vi "UI Interface.vi"(8 "error in (no error)":errorcluster, 10 "GRR Results":T1[](array[typedef]), 11 "Test Data":T2[](array[typedef])) -> (0 "error out":errorcluster)   [LabVIEW 2018, in "Result Display.lvclass"]
uses:
  Result Display.lvclass
  TestDataMgr/Typedefs/Test Data All.ctl
  TestDataMgr/Typedefs/Test Limits.ctl
  TestDataMgr/Typedefs/Test Raw Data.ctl
  Result Data Mgr/Typedefs/GRR Result.ctl
  <vilib>/Utility/error.llb/Error Cluster From Error Code.vi
  <vilib>/ErrorRing/Error Ring.xnode
  TestDataMgr/TestDataMgr.lvclass
  Result Data Mgr/Result Data Mgr.lvclass
panel:
  in  "DUT Plot Visible?  DUT# 0-N":bool[](array[boolean])
  in  "stop":bool
  out "GRR Result":T1
  out "Tester#2":dbl[][](graph)
  out "Tester#1":dbl[][](graph)
  in  "Test Items":u16(ring) items=["TXV_PS_Gmax_24p25G_V4_PhaseRange", "OS_VDD_SPI_CS", "TXV_PS_Gmax_27p5G_V0_GainDelta", "TXV_PS_Gmax_29p5G_V1_PhaseRange", "TXV_GS_Phase_Dynamic_FE_24p25G_V4", "RXV_PS_Gmax_26p5G_V1_PhaseRange", "TXV_PAE_12dBm_Pout_24p25G_V3", "TXV_PD_10dBm_Vout_24p25_V1", "TXV_PS_Gmax_24p25G_V5_GainDelta", "OS_VDD_SPI_CLK_IN", "TXV_PS_Gmax_27p5G_V0_GainRMS", "TXV_PS_Gmax_29p5G_V2_GainDelta", "TXV_GS_Gain_Gmax_COM127_FE127_24p25G_V5", "RXV_PS_Gmax_26p5G_V2_GainDelta", "TXV_PAE_12dBm_PAE_24p25G_V3", "TXV_PD_15dBm_Pout_24p25_V1", "TXV_PS_Gmax_24p25G_V5_GainRMS", "OS_VDD_SPI_DATA_IN", "TXV_PS_Gmax_27p5G_V0_PhaseRange", "TXV_PS_Gmax_29p5G_V2_GainRMS", "TXV_GS_Gain_Dynamic_COM_24p25G_V5", "RXV_PS_Gmax_26p5G_V2_GainRMS", "TXV_PAE_12dBm_Pout_24p25G_V4", "TXV_PD_15dBm_Vout_24p25_V1", "TXV_PS_Gmax_24p25G_V5_PhaseRange", "OS_VDD_SPI_DATA_OUT", "TXV_PS_Gmax_27p5G_V1_GainDelta", "TXV_PS_Gmax_29p5G_V2_PhaseRange", "TXV_GS_Gain_Dynamic_FE_24p25G_V5", "RXV_PS_Gmax_26p5G_V2_PhaseRange", "TXV_PAE_12dBm_PAE_24p25G_V4", "TXV_PD_4dBm_Pout_24p25_V2", "TXV_PS_Gmax_24p25G_V6_GainDelta", "OS_VDD_SPI_CLK_OUT", "TXV_PS_Gmax_27p5G_V1_GainRMS", "TXV_PS_Gmax_29p5G_V3_GainDelta", "TXV_GS_Phase_Dynamic_COM_24p25G_V5", "RXV_PS_Gmax_26p5G_V3_GainDelta", "TXV_PAE_12dBm_Pout_24p25G_V5", "TXV_PD_4dBm_Vout_24p25_V2", "TXV_PS_Gmax_24p25G_V6_GainRMS", "OS_VDD_DFT_MODE", "TXV_PS_Gmax_27p5G_V1_PhaseRange", "TXV_PS_Gmax_29p5G_V3_GainRMS", "TXV_GS_Phase_Dynamic_FE_24p25G_V5", "RXV_PS_Gmax_26p5G_V3_GainRMS", "TXV_PAE_12dBm_PAE_24p25G_V5", "TXV_PD_10dBm_Pout_24p25_V2", "TXV_PS_Gmax_24p25G_V6_PhaseRange", "OS_VDD_DFT_PIN1", "TXV_PS_Gmax_27p5G_V2_GainDelta", "TXV_PS_Gmax_29p5G_V3_PhaseRange", "TXV_GS_Gain_Gmax_COM127_FE127_24p25G_V6", "RXV_PS_Gmax_26p5G_V3_PhaseRange", "TXV_PAE_12dBm_Pout_24p25G_V6", "TXV_PD_10dBm_Vout_24p25_V2", "TXV_PS_Gmax_24p25G_V7_GainDelta", "OS_VDD_DFT_PIN2", "TXV_PS_Gmax_27p5G_V2_GainRMS", "TXV_PS_Gmax_29p5G_V4_GainDelta", "TXV_GS_Gain_Dynamic_COM_24p25G_V6", "RXV_PS_Gmax_26p5G_V4_GainDelta", "TXV_PAE_12dBm_PAE_24p25G_V6", "TXV_PD_15dBm_Pout_24p25_V2", "TXV_PS_Gmax_24p25G_V7_GainRMS", "OS_VDD_DFT_PIN3", "TXV_PS_Gmax_27p5G_V2_PhaseRange", "TXV_PS_Gmax_29p5G_V4_GainRMS", "TXV_GS_Gain_Dynamic_FE_24p25G_V6", "RXV_PS_Gmax_26p5G_V4_GainRMS", "TXV_PAE_12dBm_Pout_24p25G_V7", "TXV_PD_15dBm_Vout_24p25_V2", "TXV_PS_Gmax_24p25G_V7_PhaseRange", "OS_VDD_TDD_H_TRX_PIN_HV", "TXV_PS_Gmax_27p5G_V3_GainDelta", "TXV_PS_Gmax_29p5G_V4_PhaseRange", "TXV_GS_Phase_Dynamic_COM_24p25G_V6", "RXV_PS_Gmax_26p5G_V4_PhaseRange", "TXV_PAE_12dBm_PAE_24p25G_V7", "TXV_PD_4dBm_Pout_24p25_V3", "RXV_PS_Gmax_24p25G_V0_GainDelta", "OS_VDD_TDD_V_TRX_PIN_HV", "TXV_PS_Gmax_27p5G_V3_GainRMS", "TXV_PS_Gmax_29p5G_V5_GainDelta", "TXV_GS_Phase_Dynamic_FE_24p25G_V6", "RXV_PS_Gmax_26p5G_V5_GainDelta", "TXV_OIP3_Gmax_100M_OIP3_L_24p25G_V0", "TXV_PD_4dBm_Vout_24p25_V3", "RXV_PS_Gmax_24p25G_V0_GainRMS", "OS_VDD_ADC_CLK", "TXV_PS_Gmax_27p5G_V3_PhaseRange", "TXV_PS_Gmax_29p5G_V5_GainRMS", "TXV_GS_Gain_Gmax_COM127_FE127_24p25G_V7", "RXV_PS_Gmax_26p5G_V5_GainRMS", "TXV_OIP3_Gmax_100M_OIP3_H_24p25G_V0", "TXV_PD_10dBm_Pout_24p25_V3", "RXV_PS_Gmax_24p25G_V0_PhaseRange", "OS_VDD_ADC_DATA0", "TXV_PS_Gmax_27p5G_V4_GainDelta", "TXV_PS_Gmax_29p5G_V5_PhaseRange", "TXV_GS_Gain_Dynamic_COM_24p25G_V7", "RXV_PS_Gmax_26p5G_V5_PhaseRange", "TXV_OIP3_Gmax_100M_OIP3_L_24p25G_V1", "TXV_PD_10dBm_Vout_24p25_V3", "RXV_PS_Gmax_24p25G_V1_GainDelta", "OS_VDD_ADC_DATA1", "TXV_PS_Gmax_27p5G_V4_GainRMS", "TXV_PS_Gmax_29p5G_V6_GainDelta", "TXV_GS_Gain_Dynamic_FE_24p25G_V7", "RXV_PS_Gmax_26p5G_V6_GainDelta", "TXV_OIP3_Gmax_100M_OIP3_H_24p25G_V1", "TXV_PD_15dBm_Pout_24p25_V3", "RXV_PS_Gmax_24p25G_V1_GainRMS", "OS_VDD_ADC_DATA2", "TXV_PS_Gmax_27p5G_V4_PhaseRange", "TXV_PS_Gmax_29p5G_V6_GainRMS", "TXV_GS_Phase_Dynamic_COM_24p25G_V7", "RXV_PS_Gmax_26p5G_V6_GainRMS", "TXV_OIP3_Gmax_100M_OIP3_L_24p25G_V2", "TXV_PD_15dBm_Vout_24p25_V3", "RXV_PS_Gmax_24p25G_V1_PhaseRange", "OS_VDD_ADC_VALID", "TXV_PS_Gmax_27p5G_V5_GainDelta", "TXV_PS_Gmax_29p5G_V6_PhaseRange", "TXV_GS_Phase_Dynamic_FE_24p25G_V7", "RXV_PS_Gmax_26p5G_V6_PhaseRange", "TXV_OIP3_Gmax_100M_OIP3_H_24p25G_V2", "TXV_PD_4dBm_Pout_24p25_V4", "RXV_PS_Gmax_24p25G_V2_GainDelta", "OS_VDD_VTRIM_LDO_SPI_HV", "TXV_PS_Gmax_27p5G_V5_GainRMS", "TXV_PS_Gmax_29p5G_V7_GainDelta", "TXV_GS_Gain_Gmax_COM127_FE127_24p25G_ChannelDelta", "RXV_PS_Gmax_26p5G_V7_GainDelta", "TXV_OIP3_Gmax_100M_OIP3_L_24p25G_V3", "TXV_PD_4dBm_Vout_24p25_V4", "RXV_PS_Gmax_24p25G_V2_GainRMS", "OS_VDD_REXT_BG", "TXV_PS_Gmax_27p5G_V5_PhaseRange", "TXV_PS_Gmax_29p5G_V7_GainRMS", "TXV_OP1_Gmax_Pout_24p25G_V0", "RXV_PS_Gmax_26p5G_V7_GainRMS", "TXV_OIP3_Gmax_100M_OIP3_H_24p25G_V3", "TXV_PD_10dBm_Pout_24p25_V4", "RXV_PS_Gmax_24p25G_V2_PhaseRange", "OS_VDD_REXT_BG_LO", "TXV_PS_Gmax_27p5G_V6_GainDelta", "TXV_PS_Gmax_29p5G_V7_PhaseRange", "TXV_OP1_Gmax_GainCompress_24p25G_V0", "RXV_PS_Gmax_26p5G_V7_PhaseRange", "TXV_OIP3_Gmax_100M_OIP3_L_24p25G_V4", "TXV_PD_10dBm_Vout_24p25_V4", "RXV_PS_Gmax_24p25G_V3_GainDelta", "OS_VDD_DATA_IN1", "TXV_PS_Gmax_27p5G_V6_GainRMS", "RXV_PS_Gmax_29p5G_V0_GainDelta", "TXV_OP1_Gmax_Pout_24p25G_V1", "TXV_PS_Gmax_28G_V0_GainDelta", "TXV_OIP3_Gmax_100M_OIP3_H_24p25G_V4", "TXV_PD_15dBm_Pout_24p25_V4", "RXV_PS_Gmax_24p25G_V3_GainRMS", "OS_VDD_DATA_OUT1", "TXV_PS_Gmax_27p5G_V6_PhaseRange", "RXV_PS_Gmax_29p5G_V0_GainRMS", "TXV_OP1_Gmax_GainCompress_24p25G_V1", "TXV_PS_Gmax_28G_V0_GainRMS", "TXV_OIP3_Gmax_100M_OIP3_L_24p25G_V5", "TXV_PD_15dBm_Vout_24p25_V4", "RXV_PS_Gmax_24p25G_V3_PhaseRange", "OS_VDD_ASPI_BLINK_SW", "TXV_PS_Gmax_27p5G_V7_GainDelta", "RXV_PS_Gmax_29p5G_V0_PhaseRange", "TXV_OP1_Gmax_Pout_24p25G_V2", "TXV_PS_Gmax_28G_V0_PhaseRange", "TXV_OIP3_Gmax_100M_OIP3_H_24p25G_V5", "TXV_PD_4dBm_Pout_24p25_V5", "RXV_PS_Gmax_24p25G_V4_GainDelta", "OS_VSS_SPI_CS", "TXV_PS_Gmax_27p5G_V7_GainRMS", "RXV_PS_Gmax_29p5G_V1_GainDelta", "TXV_OP1_Gmax_GainCompress_24p25G_V2", "TXV_PS_Gmax_28G_V1_GainDelta", "TXV_OIP3_Gmax_100M_OIP3_L_24p25G_V6", "TXV_PD_4dBm_Vout_24p25_V5", "RXV_PS_Gmax_24p25G_V4_GainRMS", "OS_VSS_SPI_CLK_IN", "TXV_PS_Gmax_27p5G_V7_PhaseRange", "RXV_PS_Gmax_29p5G_V1_GainRMS", "TXV_OP1_Gmax_Pout_24p25G_V3", "TXV_PS_Gmax_28G_V1_GainRMS", "TXV_OIP3_Gmax_100M_OIP3_H_24p25G_V6", "TXV_PD_10dBm_Pout_24p25_V5", "RXV_PS_Gmax_24p25G_V4_PhaseRange", "OS_VSS_SPI_DATA_IN", "RXV_PS_Gmax_27p5G_V0_GainDelta", "RXV_PS_Gmax_29p5G_V1_PhaseRange", "TXV_OP1_Gmax_GainCompress_24p25G_V3", "TXV_PS_Gmax_28G_V1_PhaseRange", "TXV_OIP3_Gmax_100M_OIP3_L_24p25G_V7", "TXV_PD_10dBm_Vout_24p25_V5", "RXV_PS_Gmax_24p25G_V5_GainDelta", "OS_VSS_SPI_DATA_OUT", "RXV_PS_Gmax_27p5G_V0_GainRMS", "RXV_PS_Gmax_29p5G_V2_GainDelta", "TXV_OP1_Gmax_Pout_24p25G_V4", "TXV_PS_Gmax_28G_V2_GainDelta", "TXV_OIP3_Gmax_100M_OIP3_H_24p25G_V7", "TXV_PD_15dBm_Pout_24p25_V5", "RXV_PS_Gmax_24p25G_V5_GainRMS", "OS_VSS_SPI_CLK_OUT", "RXV_PS_Gmax_27p5G_V0_PhaseRange", "RXV_PS_Gmax_29p5G_V2_GainRMS", "TXV_OP1_Gmax_GainCompress_24p25G_V4", "TXV_PS_Gmax_28G_V2_GainRMS", "TXV_NF_Gmax_24p25_V0", "TXV_PD_15dBm_Vout_24p25_V5", "RXV_PS_Gmax_24p25G_V5_PhaseRange", "OS_VSS_DFT_MODE", "RXV_PS_Gmax_27p5G_V1_GainDelta", "RXV_PS_Gmax_29p5G_V2_PhaseRange", "TXV_OP1_Gmax_Pout_24p25G_V5", "TXV_PS_Gmax_28G_V2_PhaseRange", "TXV_NF_Gmax_24p25_V1", "TXV_PD_4dBm_Pout_24p25_V6", "RXV_PS_Gmax_24p25G_V6_GainDelta", "OS_VSS_DFT_PIN1", "RXV_PS_Gmax_27p5G_V1_GainRMS", "RXV_PS_Gmax_29p5G_V3_GainDelta", "TXV_OP1_Gmax_GainCompress_24p25G_V5", "TXV_PS_Gmax_28G_V3_GainDelta", "TXV_NF_Gmax_24p25_V2", "TXV_PD_4dBm_Vout_24p25_V6", "RXV_PS_Gmax_24p25G_V6_GainRMS", "OS_VSS_DFT_PIN2", "RXV_PS_Gmax_27p5G_V1_PhaseRange", "RXV_PS_Gmax_29p5G_V3_GainRMS", "TXV_OP1_Gmax_Pout_24p25G_V6", "TXV_PS_Gmax_28G_V3_GainRMS", "TXV_NF_Gmax_24p25_V3", "TXV_PD_10dBm_Pout_24p25_V6", "RXV_PS_Gmax_24p25G_V6_PhaseRange", "OS_VSS_DFT_PIN3", "RXV_PS_Gmax_27p5G_V2_GainDelta", "RXV_PS_Gmax_29p5G_V3_PhaseRange", "TXV_OP1_Gmax_GainCompress_24p25G_V6", "TXV_PS_Gmax_28G_V3_PhaseRange", "TXV_NF_Gmax_24p25_V4", "TXV_PD_10dBm_Vout_24p25_V6", "RXV_PS_Gmax_24p25G_V7_GainDelta", "OS_VSS_TDD_H_TRX_PIN_HV", "RXV_PS_Gmax_27p5G_V2_GainRMS", "RXV_PS_Gmax_29p5G_V4_GainDelta", "TXV_OP1_Gmax_Pout_24p25G_V7", "TXV_PS_Gmax_28G_V4_GainDelta", "TXV_NF_Gmax_24p25_V5", "TXV_PD_15dBm_Pout_24p25_V6", "RXV_PS_Gmax_24p25G_V7_GainRMS", "OS_VSS_TDD_V_TRX_PIN_HV", "RXV_PS_Gmax_27p5G_V2_PhaseRange", "RXV_PS_Gmax_29p5G_V4_GainRMS", "TXV_OP1_Gmax_GainCompress_24p25G_V7", "TXV_PS_Gmax_28G_V4_GainRMS", "TXV_NF_Gmax_24p25_V6", "TXV_PD_15dBm_Vout_24p25_V6", "RXV_PS_Gmax_24p25G_V7_PhaseRange", "OS_VSS_ADC_CLK", "RXV_PS_Gmax_27p5G_V3_GainDelta", "RXV_PS_Gmax_29p5G_V4_PhaseRange", "TXV_AMPM_12dBm_Pout_24p25G_V0", "TXV_PS_Gmax_28G_V4_PhaseRange", "TXV_NF_Gmax_24p25_V7", "TXV_PD_4dBm_Pout_24p25_V7", "TXV_PS_Gmax_25p5G_V0_GainDelta", "OS_VSS_ADC_DATA0", "RXV_PS_Gmax_27p5G_V3_GainRMS", "RXV_PS_Gmax_29p5G_V5_GainDelta", "TXV_AMAM_12dBm_GainCompress_24p25G_V0", "TXV_PS_Gmax_28G_V5_GainDelta", "TXV_NF_Gm5dB_24p25_V0", "TXV_PD_4dBm_Vout_24p25_V7", "TXV_PS_Gmax_25p5G_V0_GainRMS", "OS_VSS_ADC_DATA1", "RXV_PS_Gmax_27p5G_V3_PhaseRange", "RXV_PS_Gmax_29p5G_V5_GainRMS", "TXV_AMPM_12dBm_PhaseDelta_24p25G_V0", "TXV_PS_Gmax_28G_V5_GainRMS", "TXV_NF_Gm5dB_24p25_V1", "TXV_PD_10dBm_Pout_24p25_V7", "TXV_PS_Gmax_25p5G_V0_PhaseRange", "OS_VSS_ADC_DATA2", "RXV_PS_Gmax_27p5G_V4_GainDelta", "RXV_PS_Gmax_29p5G_V5_PhaseRange", "TXV_AMPM_12dBm_Pout_24p25G_V1", "TXV_PS_Gmax_28G_V5_PhaseRange", "TXV_NF_Gm5dB_24p25_V2", "TXV_PD_10dBm_Vout_24p25_V7", "TXV_PS_Gmax_25p5G_V1_GainDelta", "OS_VSS_ADC_VALID", "RXV_PS_Gmax_27p5G_V4_GainRMS", "RXV_PS_Gmax_29p5G_V6_GainDelta", "TXV_AMAM_12dBm_GainCompress_24p25G_V1", "TXV_PS_Gmax_28G_V6_GainDelta", "TXV_NF_Gm5dB_24p25_V3", "TXV_PD_15dBm_Pout_24p25_V7", "TXV_PS_Gmax_25p5G_V1_GainRMS", "OS_VSS_VTRIM_LDO_SPI_HV", "RXV_PS_Gmax_27p5G_V4_PhaseRange", "RXV_PS_Gmax_29p5G_V6_GainRMS", "TXV_AMPM_12dBm_PhaseDelta_24p25G_V1", "TXV_PS_Gmax_28G_V6_GainRMS", "TXV_NF_Gm5dB_24p25_V4", "TXV_PD_15dBm_Vout_24p25_V7", "TXV_PS_Gmax_25p5G_V1_PhaseRange", "OS_VSS_REXT_BG", "RXV_PS_Gmax_27p5G_V5_GainDelta", "RXV_PS_Gmax_29p5G_V6_PhaseRange", "TXV_AMPM_12dBm_Pout_24p25G_V2", "TXV_PS_Gmax_28G_V6_PhaseRange", "TXV_NF_Gm5dB_24p25_V5", "TXV_GS_Gain_Gmax_COM127_FE127_26p5G_V0", "TXV_PS_Gmax_25p5G_V2_GainDelta", "OS_VSS_REXT_BG_LO", "RXV_PS_Gmax_27p5G_V5_GainRMS", "RXV_PS_Gmax_29p5G_V7_GainDelta", "TXV_AMAM_12dBm_GainCompress_24p25G_V2", "TXV_PS_Gmax_28G_V7_GainDelta", "TXV_NF_Gm5dB_24p25_V6", "TXV_GS_Gain_Dynamic_COM_26p5G_V0", "TXV_PS_Gmax_25p5G_V2_GainRMS", "OS_VSS_DATA_IN1", "RXV_PS_Gmax_27p5G_V5_PhaseRange", "RXV_PS_Gmax_29p5G_V7_GainRMS", "TXV_AMPM_12dBm_PhaseDelta_24p25G_V2", "TXV_PS_Gmax_28G_V7_GainRMS", "TXV_NF_Gm5dB_24p25_V7", "TXV_GS_Gain_Dynamic_FE_26p5G_V0", "TXV_PS_Gmax_25p5G_V2_PhaseRange", "OS_VSS_DATA_OUT1", "RXV_PS_Gmax_27p5G_V6_GainDelta", "RXV_PS_Gmax_29p5G_V7_PhaseRange", "TXV_AMPM_12dBm_Pout_24p25G_V3", "TXV_PS_Gmax_28G_V7_PhaseRange", "TXV_NF_Gm10dB_24p25_V0", "TXV_GS_Phase_Dynamic_COM_26p5G_V0", "TXV_PS_Gmax_25p5G_V3_GainDelta", "OS_VSS_ASPI_BLINK_SW", "RXV_PS_Gmax_27p5G_V6_GainRMS", "TXV_GS_Gain_Gmax_COM127_FE127_24p25G_V0", "TXV_AMAM_12dBm_GainCompress_24p25G_V3", "RXV_PS_Gmax_28G_V0_GainDelta", "TXV_NF_Gm10dB_24p25_V1", "TXV_GS_Phase_Dynamic_FE_26p5G_V0", "TXV_PS_Gmax_25p5G_V3_GainRMS", "PS_AVCC_FE", "RXV_PS_Gmax_27p5G_V6_PhaseRange", "TXV_GS_Gain_Dynamic_COM_24p25G_V0", "TXV_AMPM_12dBm_PhaseDelta_24p25G_V3", "RXV_PS_Gmax_28G_V0_GainRMS", "TXV_NF_Gm10dB_24p25_V2", "TXV_GS_Gain_Gmax_COM127_FE127_26p5G_V1", "TXV_PS_Gmax_25p5G_V3_PhaseRange", "PS_AVCC_PA", "RXV_PS_Gmax_27p5G_V7_GainDelta", "TXV_GS_Gain_Dynamic_FE_24p25G_V0", "TXV_AMPM_12dBm_Pout_24p25G_V4", "RXV_PS_Gmax_28G_V0_PhaseRange", "TXV_NF_Gm10dB_24p25_V3", "TXV_GS_Gain_Dynamic_COM_26p5G_V1", "TXV_PS_Gmax_25p5G_V4_GainDelta", "DC_ICT_AVCC_FE", "RXV_PS_Gmax_27p5G_V7_GainRMS", "TXV_GS_Phase_Dynamic_COM_24p25G_V0", "TXV_AMAM_12dBm_GainCompress_24p25G_V4", "RXV_PS_Gmax_28G_V1_GainDelta", "TXV_NF_Gm10dB_24p25_V4", "TXV_GS_Gain_Dynamic_FE_26p5G_V1", "TXV_PS_Gmax_25p5G_V4_GainRMS", "DC_ICT_AVCC_PA", "RXV_PS_Gmax_27p5G_V7_PhaseRange", "TXV_GS_Phase_Dynamic_FE_24p25G_V0", "TXV_AMPM_12dBm_PhaseDelta_24p25G_V4", "RXV_PS_Gmax_28G_V1_GainRMS", "TXV_NF_Gm10dB_24p25_V5", "TXV_GS_Phase_Dynamic_COM_26p5G_V1", "TXV_PS_Gmax_25p5G_V4_PhaseRange", "DC_IIH_SPI_CS", "TXV_PS_Gmax_26p5G_V0_GainDelta", "TXV_GS_Gain_Gmax_COM127_FE127_24p25G_V1", "TXV_AMPM_12dBm_Pout_24p25G_V5", "RXV_PS_Gmax_28G_V1_PhaseRange", "TXV_NF_Gm10dB_24p25_V6", "TXV_GS_Phase_Dynamic_FE_26p5G_V1", "TXV_PS_Gmax_25p5G_V5_GainDelta", "DC_IIH_SPI_CLK_IN", "TXV_PS_Gmax_26p5G_V0_GainRMS", "TXV_GS_Gain_Dynamic_COM_24p25G_V1", "TXV_AMAM_12dBm_GainCompress_24p25G_V5", "RXV_PS_Gmax_28G_V2_GainDelta", "TXV_NF_Gm10dB_24p25_V7", "TXV_GS_Gain_Gmax_COM127_FE127_26p5G_V2", "TXV_PS_Gmax_25p5G_V5_GainRMS", "DC_IIH_SPI_DATA_IN", "TXV_PS_Gmax_26p5G_V0_PhaseRange", "TXV_GS_Gain_Dynamic_FE_24p25G_V1", "TXV_AMPM_12dBm_PhaseDelta_24p25G_V5", "RXV_PS_Gmax_28G_V2_GainRMS", "TXV_PD_4dBm_Pout_24p25_V0", "TXV_GS_Gain_Dynamic_COM_26p5G_V2", "TXV_PS_Gmax_25p5G_V5_PhaseRange", "DC_IIL_SPI_CS", "TXV_PS_Gmax_26p5G_V1_GainDelta", "TXV_GS_Phase_Dynamic_COM_24p25G_V1", "TXV_AMPM_12dBm_Pout_24p25G_V6", "RXV_PS_Gmax_28G_V2_PhaseRange", "TXV_PD_4dBm_Vout_24p25_V0", "TXV_GS_Gain_Dynamic_FE_26p5G_V2", "TXV_PS_Gmax_25p5G_V6_GainDelta", "DC_IIL_SPI_CLK_IN", "TXV_PS_Gmax_26p5G_V1_GainRMS", "TXV_GS_Phase_Dynamic_FE_24p25G_V1", "TXV_AMAM_12dBm_GainCompress_24p25G_V6", "RXV_PS_Gmax_28G_V3_GainDelta", "TXV_PD_10dBm_Pout_24p25_V0", "TXV_GS_Phase_Dynamic_COM_26p5G_V2", "TXV_PS_Gmax_25p5G_V6_GainRMS", "DC_IIL_SPI_DATA_IN", "TXV_PS_Gmax_26p5G_V1_PhaseRange", "TXV_GS_Gain_Gmax_COM127_FE127_24p25G_V2", "TXV_AMPM_12dBm_PhaseDelta_24p25G_V6", "RXV_PS_Gmax_28G_V3_GainRMS", "TXV_PD_10dBm_Vout_24p25_V0", "TXV_GS_Phase_Dynamic_FE_26p5G_V2", "TXV_PS_Gmax_25p5G_V6_PhaseRange", "DC_BandGap", "TXV_PS_Gmax_26p5G_V2_GainDelta", "TXV_GS_Gain_Dynamic_COM_24p25G_V2", "TXV_AMPM_12dBm_Pout_24p25G_V7", "RXV_PS_Gmax_28G_V3_PhaseRange", "TXV_PD_15dBm_Pout_24p25_V0", "TXV_GS_Gain_Gmax_COM127_FE127_26p5G_V3", "TXV_PS_Gmax_25p5G_V7_GainDelta", "BangGap_Trim_Default_Voltage", "TXV_PS_Gmax_26p5G_V2_GainRMS", "TXV_GS_Gain_Dynamic_FE_24p25G_V2", "TXV_AMAM_12dBm_GainCompress_24p25G_V7", "RXV_PS_Gmax_28G_V4_GainDelta", "TXV_PD_15dBm_Vout_24p25_V0", "TXV_GS_Gain_Dynamic_COM_26p5G_V3", "TXV_PS_Gmax_25p5G_V7_GainRMS", "BangGap_Trim_Voltage", "TXV_PS_Gmax_26p5G_V2_PhaseRange", "TXV_GS_Phase_Dynamic_COM_24p25G_V2", "TXV_AMPM_12dBm_PhaseDelta_24p25G_V7", "RXV_PS_Gmax_28G_V4_GainRMS", "TXV_PD_4dBm_Pout_24p25_V1", "TXV_GS_Gain_Dynamic_FE_26p5G_V3", "TXV_PS_Gmax_25p5G_V7_PhaseRange", "DC_TXV_Standby_AVCC_FE", "TXV_PS_Gmax_26p5G_V3_GainDelta", "TXV_GS_Phase_Dynamic_FE_24p25G_V2", "TXV_PAE_12dBm_Pout_24p25G_V0", "RXV_PS_Gmax_28G_V4_PhaseRange", "TXV_PD_4dBm_Vout_24p25_V1", "TXV_GS_Phase_Dynamic_COM_26p5G_V3", "RXV_PS_Gmax_25p5G_V0_GainDelta", "DC_TXV_Standby_AVCC_PA", "TXV_PS_Gmax_26p5G_V3_GainRMS", "TXV_GS_Gain_Gmax_COM127_FE127_24p25G_V3", "TXV_PAE_12dBm_PAE_24p25G_V0", "RXV_PS_Gmax_28G_V5_GainDelta", "TXV_PD_10dBm_Pout_24p25_V1", "TXV_GS_Phase_Dynamic_FE_26p5G_V3", "RXV_PS_Gmax_25p5G_V0_GainRMS", "DC_TXV_Idle_AVCC_FE", "TXV_PS_Gmax_26p5G_V3_PhaseRange", "TXV_GS_Gain_Dynamic_COM_24p25G_V3", "TXV_PAE_12dBm_Pout_24p25G_V1", "TXV_AMPM_12dBm_PhaseDelta_26p5G_V3", "RXV_PS_Gmax_28G_V5_GainRMS", "TXV_GS_Gain_Gmax_COM127_FE127_26p5G_V4", "RXV_PS_Gmax_25p5G_V0_PhaseRange", "DC_TXV_Idle_AVCC_PA", "TXV_PS_Gmax_26p5G_V4_GainDelta", "TXV_GS_Gain_Dynamic_FE_24p25G_V3", "TXV_PAE_12dBm_PAE_24p25G_V1", "TXV_AMPM_12dBm_Pout_26p5G_V4", "RXV_PS_Gmax_28G_V5_PhaseRange", "TXV_GS_Gain_Dynamic_COM_26p5G_V4", "RXV_PS_Gmax_25p5G_V1_GainDelta", "DC_TXV_ON_AVCC_FE", "TXV_PS_Gmax_26p5G_V4_GainRMS", "TXV_GS_Phase_Dynamic_COM_24p25G_V3", "TXV_PAE_12dBm_Pout_24p25G_V2", "TXV_AMAM_12dBm_GainCompress_26p5G_V4", "RXV_PS_Gmax_28G_V6_GainDelta", "TXV_GS_Gain_Dynamic_FE_26p5G_V4", "RXV_PS_Gmax_25p5G_V1_GainRMS", "DC_TXV_ON_AVCC_PA", "TXV_PS_Gmax_26p5G_V4_PhaseRange", "TXV_GS_Phase_Dynamic_FE_24p25G_V3", "TXV_PAE_12dBm_PAE_24p25G_V2", "TXV_AMPM_12dBm_PhaseDelta_26p5G_V4", "RXV_PS_Gmax_28G_V6_GainRMS", "TXV_GS_Phase_Dynamic_COM_26p5G_V4", "RXV_PS_Gmax_25p5G_V1_PhaseRange", "DC_RXV_Standby_AVCC_FE", "TXV_PS_Gmax_26p5G_V5_GainDelta", "TXV_GS_Gain_Gmax_COM127_FE127_24p25G_V4", "TXV_NF_Gmax_26p5_V4", "TXV_AMPM_12dBm_Pout_26p5G_V5", "RXV_PS_Gmax_28G_V6_PhaseRange", "TXV_GS_Phase_Dynamic_FE_26p5G_V4", "RXV_PS_Gmax_25p5G_V2_GainDelta", "DC_RXV_Standby_AVCC_PA", "TXV_PS_Gmax_26p5G_V5_GainRMS", "TXV_GS_Gain_Dynamic_COM_24p25G_V4", "TXV_NF_Gmax_26p5_V5", "TXV_AMAM_12dBm_GainCompress_26p5G_V5", "RXV_PS_Gmax_28G_V7_GainDelta", "TXV_GS_Gain_Gmax_COM127_FE127_26p5G_V5", "RXV_PS_Gmax_25p5G_V2_GainRMS", "DC_RXV_Idle_AVCC_FE", "TXV_PS_Gmax_26p5G_V5_PhaseRange", "TXV_GS_Gain_Dynamic_FE_24p25G_V4", "TXV_NF_Gmax_26p5_V6", "TXV_AMPM_12dBm_PhaseDelta_26p5G_V5", "RXV_PS_Gmax_28G_V7_GainRMS", "TXV_GS_Gain_Dynamic_COM_26p5G_V5", "RXV_PS_Gmax_25p5G_V2_PhaseRange", "DC_RXV_Idle_AVCC_PA", "TXV_PS_Gmax_26p5G_V6_GainDelta", "TXV_GS_Phase_Dynamic_COM_24p25G_V4", "TXV_NF_Gmax_26p5_V7", "TXV_AMPM_12dBm_Pout_26p5G_V6", "RXV_PS_Gmax_28G_V7_PhaseRange", "TXV_GS_Gain_Dynamic_FE_26p5G_V5", "RXV_PS_Gmax_25p5G_V3_GainDelta", "DC_RXV_ON_AVCC_FE", "TXV_PS_Gmax_26p5G_V6_GainRMS", "TXV_PD_10dBm_Pout_26p5_V4", "TXV_NF_Gm5dB_26p5_V0", "TXV_AMAM_12dBm_GainCompress_26p5G_V6", "TXV_PS_Gmax_29p5G_V0_GainDelta", "TXV_GS_Phase_Dynamic_COM_26p5G_V5", "RXV_PS_Gmax_25p5G_V3_GainRMS", "DC_RXV_ON_AVCC_PA", "TXV_PS_Gmax_26p5G_V6_PhaseRange", "TXV_PD_10dBm_Vout_26p5_V4", "TXV_NF_Gm5dB_26p5_V1", "TXV_AMPM_12dBm_PhaseDelta_26p5G_V6", "TXV_PS_Gmax_29p5G_V0_GainRMS", "TXV_GS_Phase_Dynamic_FE_26p5G_V5", "RXV_PS_Gmax_25p5G_V3_PhaseRange", "DC_IF_TXV_ON_AVCC_FE", "TXV_PS_Gmax_26p5G_V7_GainDelta", "TXV_PD_15dBm_Pout_26p5_V4", "TXV_NF_Gm5dB_26p5_V2", "TXV_AMPM_12dBm_Pout_26p5G_V7", "TXV_PS_Gmax_29p5G_V0_PhaseRange", "TXV_GS_Gain_Gmax_COM127_FE127_26p5G_V6", "RXV_PS_Gmax_25p5G_V4_GainDelta", "DC_IF_TXV_ON_AVCC_PA", "TXV_PS_Gmax_26p5G_V7_GainRMS", "TXV_PD_15dBm_Vout_26p5_V4", "TXV_NF_Gm5dB_26p5_V3", "TXV_AMAM_12dBm_GainCompress_26p5G_V7", "TXV_PS_Gmax_29p5G_V1_GainDelta", "TXV_GS_Gain_Dynamic_COM_26p5G_V6", "RXV_PS_Gmax_25p5G_V4_GainRMS", "DC_IF_RXV_ON_AVCC_FE", "TXV_PS_Gmax_26p5G_V7_PhaseRange", "TXV_PD_4dBm_Pout_26p5_V5", "TXV_NF_Gm5dB_26p5_V4", "TXV_AMPM_12dBm_PhaseDelta_26p5G_V7", "TXV_PS_Gmax_29p5G_V1_GainRMS", "TXV_GS_Gain_Dynamic_FE_26p5G_V6", "RXV_PS_Gmax_25p5G_V4_PhaseRange", "DC_IF_RXV_ON_AVCC_PA", "RXV_PS_Gmax_26p5G_V0_GainDelta", "TXV_PD_4dBm_Vout_26p5_V5", "TXV_NF_Gm5dB_26p5_V5", "TXV_PAE_12dBm_Pout_26p5G_V0", "TXV_GS_Gain_Dynamic_COM_28G_V4", "TXV_GS_Phase_Dynamic_COM_26p5G_V6", "RXV_PS_Gmax_25p5G_V5_GainDelta", "TXV_PS_Gmax_24p25G_V0_GainDelta", "RXV_PS_Gmax_26p5G_V0_GainRMS", "TXV_PD_10dBm_Pout_26p5_V5", "TXV_NF_Gm5dB_26p5_V6", "TXV_PAE_12dBm_PAE_26p5G_V0", "TXV_GS_Gain_Dynamic_FE_28G_V4", "TXV_GS_Phase_Dynamic_FE_26p5G_V6", "RXV_PS_Gmax_25p5G_V5_GainRMS", "TXV_PS_Gmax_24p25G_V0_GainRMS", "RXV_PS_Gmax_26p5G_V0_PhaseRange", "TXV_PD_10dBm_Vout_26p5_V5", "TXV_NF_Gm5dB_26p5_V7", "TXV_PAE_12dBm_Pout_26p5G_V1", "TXV_GS_Phase_Dynamic_COM_28G_V4", "TXV_GS_Gain_Gmax_COM127_FE127_26p5G_V7", "RXV_PS_Gmax_25p5G_V5_PhaseRange", "TXV_PS_Gmax_24p25G_V0_PhaseRange", "RXV_PS_Gmax_26p5G_V1_GainDelta", "TXV_PD_15dBm_Pout_26p5_V5", "TXV_NF_Gm10dB_26p5_V0", "TXV_PAE_12dBm_PAE_26p5G_V1", "TXV_GS_Phase_Dynamic_FE_28G_V4", "TXV_GS_Gain_Dynamic_COM_26p5G_V7", "RXV_PS_Gmax_25p5G_V6_GainDelta", "TXV_PS_Gmax_24p25G_V1_GainDelta", "RXV_PS_Gmax_26p5G_V1_GainRMS", "TXV_PD_15dBm_Vout_26p5_V5", "TXV_NF_Gm10dB_26p5_V1", "TXV_PAE_12dBm_Pout_26p5G_V2", "TXV_GS_Gain_Gmax_COM127_FE127_28G_V5", "TXV_GS_Gain_Dynamic_FE_26p5G_V7", "RXV_PS_Gmax_25p5G_V6_GainRMS", "TXV_PS_Gmax_24p25G_V1_GainRMS", "TXV_AMAM_12dBm_GainCompress_28G_V1", "TXV_PD_4dBm_Pout_26p5_V6", "TXV_NF_Gm10dB_26p5_V2", "TXV_PAE_12dBm_PAE_26p5G_V2", "TXV_GS_Gain_Dynamic_COM_28G_V5", "TXV_GS_Phase_Dynamic_COM_26p5G_V7", "RXV_PS_Gmax_25p5G_V6_PhaseRange", "TXV_PS_Gmax_24p25G_V1_PhaseRange", "TXV_AMPM_12dBm_PhaseDelta_28G_V1", "TXV_PD_4dBm_Vout_26p5_V6", "TXV_NF_Gm10dB_26p5_V3", "TXV_PAE_12dBm_Pout_26p5G_V3", "TXV_GS_Gain_Dynamic_FE_28G_V5", "TXV_GS_Phase_Dynamic_FE_26p5G_V7", "RXV_PS_Gmax_25p5G_V7_GainDelta", "TXV_PS_Gmax_24p25G_V2_GainDelta", "TXV_AMPM_12dBm_Pout_28G_V2", "TXV_PD_10dBm_Pout_26p5_V6", "TXV_NF_Gm10dB_26p5_V4", "TXV_PAE_12dBm_PAE_26p5G_V3", "TXV_GS_Phase_Dynamic_COM_28G_V5", "TXV_GS_Gain_Gmax_COM127_FE127_26p5G_ChannelDelta", "RXV_PS_Gmax_25p5G_V7_GainRMS", "TXV_PS_Gmax_24p25G_V2_GainRMS", "TXV_AMAM_12dBm_GainCompress_28G_V2", "TXV_PD_10dBm_Vout_26p5_V6", "TXV_NF_Gm10dB_26p5_V5", "TXV_PAE_12dBm_Pout_26p5G_V4", "TXV_GS_Phase_Dynamic_FE_28G_V5", "TXV_OP1_Gmax_Pout_26p5G_V0", "RXV_PS_Gmax_25p5G_V7_PhaseRange", "TXV_PS_Gmax_24p25G_V2_PhaseRange", "TXV_AMPM_12dBm_PhaseDelta_28G_V2", "TXV_PD_15dBm_Pout_26p5_V6", "TXV_NF_Gm10dB_26p5_V6", "TXV_PAE_12dBm_PAE_26p5G_V4", "TXV_GS_Gain_Gmax_COM127_FE127_28G_V6", "TXV_OP1_Gmax_GainCompress_26p5G_V0", "TXV_OIP3_Gmax_100M_OIP3_L_28G_V1", "TXV_PS_Gmax_24p25G_V3_GainDelta", "TXV_AMPM_12dBm_Pout_28G_V3", "TXV_PD_15dBm_Vout_26p5_V6", "TXV_NF_Gm10dB_26p5_V7", "TXV_PAE_12dBm_Pout_26p5G_V5", "TXV_GS_Gain_Dynamic_COM_28G_V6", "TXV_OP1_Gmax_Pout_26p5G_V1", "TXV_OIP3_Gmax_100M_OIP3_H_28G_V1", "TXV_PS_Gmax_24p25G_V3_GainRMS", "TXV_AMAM_12dBm_GainCompress_28G_V3", "TXV_PD_4dBm_Pout_26p5_V7", "TXV_PD_4dBm_Pout_26p5_V0", "TXV_PAE_12dBm_PAE_26p5G_V5", "TXV_GS_Gain_Dynamic_FE_28G_V6", "TXV_OP1_Gmax_GainCompress_26p5G_V1", "TXV_OIP3_Gmax_100M_OIP3_L_28G_V2", "TXV_PS_Gmax_24p25G_V3_PhaseRange", "TXV_AMPM_12dBm_PhaseDelta_28G_V3", "TXV_PD_4dBm_Vout_26p5_V7", "TXV_PD_4dBm_Vout_26p5_V0", "TXV_PAE_12dBm_Pout_26p5G_V6", "TXV_GS_Phase_Dynamic_COM_28G_V6", "TXV_OP1_Gmax_Pout_26p5G_V2", "TXV_OIP3_Gmax_100M_OIP3_H_28G_V2", "TXV_PS_Gmax_24p25G_V4_GainDelta", "TXV_AMPM_12dBm_Pout_28G_V4", "TXV_PD_10dBm_Pout_26p5_V7", "TXV_PD_10dBm_Pout_26p5_V0", "TXV_PAE_12dBm_PAE_26p5G_V6", "TXV_GS_Phase_Dynamic_FE_28G_V6", "TXV_OP1_Gmax_GainCompress_26p5G_V2", "TXV_OIP3_Gmax_100M_OIP3_L_28G_V3", "TXV_PS_Gmax_24p25G_V4_GainRMS", "TXV_AMAM_12dBm_GainCompress_28G_V4", "TXV_PD_10dBm_Vout_26p5_V7", "TXV_PD_10dBm_Vout_26p5_V0", "TXV_PAE_12dBm_Pout_26p5G_V7", "TXV_GS_Gain_Gmax_COM127_FE127_28G_V7", "TXV_OP1_Gmax_Pout_26p5G_V3", "TXV_OIP3_Gmax_100M_OIP3_H_28G_V3", "TXV_NF_Gm10dB_28G_V5", "TXV_AMPM_12dBm_PhaseDelta_28G_V4", "TXV_PD_15dBm_Pout_26p5_V7", "TXV_PD_15dBm_Pout_26p5_V0", "TXV_PAE_12dBm_PAE_26p5G_V7", "TXV_GS_Gain_Dynamic_COM_28G_V7", "TXV_OP1_Gmax_GainCompress_26p5G_V3", "TXV_OIP3_Gmax_100M_OIP3_L_28G_V4", "TXV_NF_Gm10dB_28G_V6", "TXV_AMPM_12dBm_Pout_28G_V5", "TXV_PD_15dBm_Vout_26p5_V7", "TXV_PD_15dBm_Vout_26p5_V0", "TXV_OIP3_Gmax_100M_OIP3_L_26p5G_V0", "TXV_GS_Gain_Dynamic_FE_28G_V7", "TXV_OP1_Gmax_Pout_26p5G_V4", "TXV_OIP3_Gmax_100M_OIP3_H_28G_V4", "TXV_NF_Gm10dB_28G_V7", "TXV_AMAM_12dBm_GainCompress_28G_V5", "TXV_GS_Gain_Gmax_COM127_FE127_28G_V0", "TXV_PD_4dBm_Pout_26p5_V1", "TXV_OIP3_Gmax_100M_OIP3_H_26p5G_V0", "TXV_GS_Phase_Dynamic_COM_28G_V7", "TXV_OP1_Gmax_GainCompress_26p5G_V4", "TXV_OIP3_Gmax_100M_OIP3_L_28G_V5", "TXV_PD_4dBm_Pout_28G_V0", "TXV_AMPM_12dBm_PhaseDelta_28G_V5", "TXV_GS_Gain_Dynamic_COM_28G_V0", "TXV_PD_4dBm_Vout_26p5_V1", "TXV_OIP3_Gmax_100M_OIP3_L_26p5G_V1", "TXV_GS_Phase_Dynamic_FE_28G_V7", "TXV_OP1_Gmax_Pout_26p5G_V5", "TXV_OIP3_Gmax_100M_OIP3_H_28G_V5", "TXV_PD_4dBm_Vout_28G_V0", "TXV_AMPM_12dBm_Pout_28G_V6", "TXV_GS_Gain_Dynamic_FE_28G_V0", "TXV_PD_10dBm_Pout_26p5_V1", "TXV_OIP3_Gmax_100M_OIP3_H_26p5G_V1", "TXV_GS_Gain_Gmax_COM127_FE127_28G_ChannelDelta", "TXV_OP1_Gmax_GainCompress_26p5G_V5", "TXV_OIP3_Gmax_100M_OIP3_L_28G_V6", "TXV_PD_10dBm_Pout_28G_V0", "TXV_AMAM_12dBm_GainCompress_28G_V6", "TXV_GS_Phase_Dynamic_COM_28G_V0", "TXV_PD_10dBm_Vout_26p5_V1", "TXV_OIP3_Gmax_100M_OIP3_L_26p5G_V2", "TXV_OP1_Gmax_Pout_28G_V0", "TXV_OP1_Gmax_Pout_26p5G_V6", "TXV_OIP3_Gmax_100M_OIP3_H_28G_V6", "TXV_PD_10dBm_Vout_28G_V0", "TXV_AMPM_12dBm_PhaseDelta_28G_V6", "TXV_GS_Phase_Dynamic_FE_28G_V0", "TXV_PD_15dBm_Pout_26p5_V1", "TXV_OIP3_Gmax_100M_OIP3_H_26p5G_V2", "TXV_OP1_Gmax_GainCompress_28G_V0", "TXV_OP1_Gmax_GainCompress_26p5G_V6", "TXV_OIP3_Gmax_100M_OIP3_L_28G_V7", "TXV_PD_15dBm_Pout_28G_V0", "TXV_AMPM_12dBm_Pout_28G_V7", "TXV_GS_Gain_Gmax_COM127_FE127_28G_V1", "TXV_PD_15dBm_Vout_26p5_V1", "TXV_OIP3_Gmax_100M_OIP3_L_26p5G_V3", "TXV_OP1_Gmax_Pout_28G_V1", "TXV_OP1_Gmax_Pout_26p5G_V7", "TXV_OIP3_Gmax_100M_OIP3_H_28G_V7", "TXV_PD_15dBm_Vout_28G_V0", "TXV_AMAM_12dBm_GainCompress_28G_V7", "TXV_GS_Gain_Dynamic_COM_28G_V1", "TXV_PD_4dBm_Pout_26p5_V2", "TXV_OIP3_Gmax_100M_OIP3_H_26p5G_V3", "TXV_OP1_Gmax_GainCompress_28G_V1", "TXV_OP1_Gmax_GainCompress_26p5G_V7", "TXV_NF_Gmax_28G_V0", "TXV_PD_4dBm_Pout_28G_V1", "TXV_AMPM_12dBm_PhaseDelta_28G_V7", "TXV_GS_Gain_Dynamic_FE_28G_V1", "TXV_PD_4dBm_Vout_26p5_V2", "TXV_OIP3_Gmax_100M_OIP3_L_26p5G_V4", "TXV_OP1_Gmax_Pout_28G_V2", "TXV_AMPM_12dBm_Pout_26p5G_V0", "TXV_NF_Gmax_28G_V1", "TXV_PD_4dBm_Vout_28G_V1", "TXV_PAE_12dBm_Pout_28G_V0", "TXV_GS_Phase_Dynamic_COM_28G_V1", "TXV_PD_10dBm_Pout_26p5_V2", "TXV_OIP3_Gmax_100M_OIP3_H_26p5G_V4", "TXV_OP1_Gmax_GainCompress_28G_V2", "TXV_AMAM_12dBm_GainCompress_26p5G_V0", "TXV_NF_Gmax_28G_V2", "TXV_PD_10dBm_Pout_28G_V1", "TXV_PAE_12dBm_PAE_28G_V0", "TXV_GS_Phase_Dynamic_FE_28G_V1", "TXV_PD_10dBm_Vout_26p5_V2", "TXV_OIP3_Gmax_100M_OIP3_L_26p5G_V5", "TXV_OP1_Gmax_Pout_28G_V3", "TXV_AMPM_12dBm_PhaseDelta_26p5G_V0", "TXV_NF_Gmax_28G_V3", "TXV_PD_10dBm_Vout_28G_V1", "TXV_PAE_12dBm_Pout_28G_V1", "TXV_GS_Gain_Gmax_COM127_FE127_28G_V2", "TXV_PD_15dBm_Pout_26p5_V2", "TXV_OIP3_Gmax_100M_OIP3_H_26p5G_V5", "TXV_OP1_Gmax_GainCompress_28G_V3", "TXV_AMPM_12dBm_Pout_26p5G_V1", "TXV_NF_Gmax_28G_V4", "TXV_PD_15dBm_Pout_28G_V1", "TXV_PAE_12dBm_PAE_28G_V1", "TXV_GS_Gain_Dynamic_COM_28G_V2", "TXV_PD_15dBm_Vout_26p5_V2", "TXV_OIP3_Gmax_100M_OIP3_L_26p5G_V6", "TXV_OP1_Gmax_Pout_28G_V4", "TXV_AMAM_12dBm_GainCompress_26p5G_V1", "TXV_NF_Gmax_28G_V5", "TXV_PD_15dBm_Vout_28G_V1", "TXV_PAE_12dBm_Pout_28G_V2", "TXV_GS_Gain_Dynamic_FE_28G_V2", "TXV_PD_4dBm_Pout_26p5_V3", "TXV_OIP3_Gmax_100M_OIP3_H_26p5G_V6", "TXV_OP1_Gmax_GainCompress_28G_V4", "TXV_AMPM_12dBm_PhaseDelta_26p5G_V1", "TXV_NF_Gmax_28G_V6", "TXV_PD_4dBm_Pout_28G_V2", "TXV_PAE_12dBm_PAE_28G_V2", "TXV_GS_Phase_Dynamic_COM_28G_V2", "TXV_PD_4dBm_Vout_26p5_V3", "TXV_OIP3_Gmax_100M_OIP3_L_26p5G_V7", "TXV_OP1_Gmax_Pout_28G_V5", "TXV_AMPM_12dBm_Pout_26p5G_V2", "TXV_NF_Gmax_28G_V7", "TXV_PD_4dBm_Vout_28G_V2", "TXV_PAE_12dBm_Pout_28G_V3", "TXV_GS_Phase_Dynamic_FE_28G_V2", "TXV_PD_10dBm_Pout_26p5_V3", "TXV_OIP3_Gmax_100M_OIP3_H_26p5G_V7", "TXV_OP1_Gmax_GainCompress_28G_V5", "TXV_AMAM_12dBm_GainCompress_26p5G_V2", "TXV_NF_Gm5dB_28G_V0", "TXV_PD_10dBm_Pout_28G_V2", "TXV_PAE_12dBm_PAE_28G_V3", "TXV_GS_Gain_Gmax_COM127_FE127_28G_V3", "TXV_PD_10dBm_Vout_26p5_V3", "TXV_NF_Gmax_26p5_V0", "TXV_OP1_Gmax_Pout_28G_V6", "TXV_AMPM_12dBm_PhaseDelta_26p5G_V2", "TXV_NF_Gm5dB_28G_V1", "TXV_PD_10dBm_Vout_28G_V2", "TXV_PAE_12dBm_Pout_28G_V4", "TXV_GS_Gain_Dynamic_COM_28G_V3", "TXV_PD_15dBm_Pout_26p5_V3", "TXV_NF_Gmax_26p5_V1", "TXV_OP1_Gmax_GainCompress_28G_V6", "TXV_AMPM_12dBm_Pout_26p5G_V3", "TXV_NF_Gm5dB_28G_V2", "TXV_PD_15dBm_Pout_28G_V2", "TXV_PAE_12dBm_PAE_28G_V4", "TXV_GS_Gain_Dynamic_FE_28G_V3", "TXV_PD_15dBm_Vout_26p5_V3", "TXV_NF_Gmax_26p5_V2", "TXV_OP1_Gmax_Pout_28G_V7", "TXV_AMAM_12dBm_GainCompress_26p5G_V3", "TXV_NF_Gm5dB_28G_V3", "TXV_PD_15dBm_Vout_28G_V2", "TXV_PAE_12dBm_Pout_28G_V5", "TXV_GS_Phase_Dynamic_COM_28G_V3", "TXV_PD_4dBm_Pout_26p5_V4", "TXV_NF_Gmax_26p5_V3", "TXV_OP1_Gmax_GainCompress_28G_V7", "TXV_PD_4dBm_Pout_28G_V5", "TXV_NF_Gm5dB_28G_V4", "TXV_PD_4dBm_Pout_28G_V3", "TXV_PAE_12dBm_PAE_28G_V5", "TXV_GS_Phase_Dynamic_FE_28G_V3", "TXV_PD_4dBm_Vout_26p5_V4", "TXV_GS_Phase_Dynamic_COM_29p5G_V2", "TXV_AMPM_12dBm_Pout_28G_V0", "TXV_PD_4dBm_Vout_28G_V5", "TXV_NF_Gm5dB_28G_V5", "TXV_PD_4dBm_Vout_28G_V3", "TXV_PAE_12dBm_Pout_28G_V6", "TXV_GS_Gain_Gmax_COM127_FE127_28G_V4", "TXV_OP1_Gmax_GainCompress_29p5G_V0", "TXV_GS_Phase_Dynamic_FE_29p5G_V2", "TXV_AMAM_12dBm_GainCompress_28G_V0", "TXV_PD_10dBm_Pout_28G_V5", "TXV_NF_Gm5dB_28G_V6", "TXV_PD_10dBm_Pout_28G_V3", "TXV_PAE_12dBm_PAE_28G_V6", "TXV_AMPM_12dBm_Pout_29p5G_V4", "TXV_OP1_Gmax_Pout_29p5G_V1", "TXV_GS_Gain_Gmax_COM127_FE127_29p5G_V3", "TXV_AMPM_12dBm_PhaseDelta_28G_V0", "TXV_PD_10dBm_Vout_28G_V5", "TXV_NF_Gm5dB_28G_V7", "TXV_PD_10dBm_Vout_28G_V3", "TXV_PAE_12dBm_Pout_28G_V7", "TXV_AMAM_12dBm_GainCompress_29p5G_V4", "TXV_OP1_Gmax_GainCompress_29p5G_V1", "TXV_GS_Gain_Dynamic_COM_29p5G_V3", "TXV_AMPM_12dBm_Pout_28G_V1", "TXV_PD_15dBm_Pout_28G_V5", "TXV_NF_Gm10dB_28G_V0", "TXV_PD_15dBm_Pout_28G_V3", "TXV_PAE_12dBm_PAE_28G_V7", "TXV_AMPM_12dBm_PhaseDelta_29p5G_V4", "TXV_OP1_Gmax_Pout_29p5G_V2", "TXV_GS_Gain_Dynamic_FE_29p5G_V3", "TXV_PAE_12dBm_Pout_29p5G_V7", "TXV_PD_15dBm_Vout_28G_V5", "TXV_NF_Gm10dB_28G_V1", "TXV_PD_15dBm_Vout_28G_V3", "TXV_OIP3_Gmax_100M_OIP3_L_28G_V0", "TXV_AMPM_12dBm_Pout_29p5G_V5", "TXV_OP1_Gmax_GainCompress_29p5G_V2", "TXV_GS_Phase_Dynamic_COM_29p5G_V3", "TXV_PAE_12dBm_PAE_29p5G_V7", "TXV_PD_4dBm_Pout_28G_V6", "TXV_NF_Gm10dB_28G_V2", "TXV_PD_4dBm_Pout_28G_V4", "TXV_OIP3_Gmax_100M_OIP3_H_28G_V0", "TXV_AMAM_12dBm_GainCompress_29p5G_V5", "TXV_OP1_Gmax_Pout_29p5G_V3", "TXV_GS_Phase_Dynamic_FE_29p5G_V3", "TXV_OIP3_Gmax_100M_OIP3_L_29p5G_V0", "TXV_PD_4dBm_Vout_28G_V6", "TXV_NF_Gm10dB_28G_V3", "TXV_PD_4dBm_Vout_28G_V4", "TXV_NF_Gmax_29p5_V6", "TXV_AMPM_12dBm_PhaseDelta_29p5G_V5", "TXV_OP1_Gmax_GainCompress_29p5G_V3", "TXV_GS_Gain_Gmax_COM127_FE127_29p5G_V4", "TXV_OIP3_Gmax_100M_OIP3_H_29p5G_V0", "TXV_PD_10dBm_Pout_28G_V6", "TXV_NF_Gm10dB_28G_V4", "TXV_PD_10dBm_Pout_28G_V4", "TXV_NF_Gmax_29p5_V7", "TXV_AMPM_12dBm_Pout_29p5G_V6", "TXV_OP1_Gmax_Pout_29p5G_V4", "TXV_GS_Gain_Dynamic_COM_29p5G_V4", "TXV_OIP3_Gmax_100M_OIP3_L_29p5G_V1", "TXV_PD_10dBm_Vout_28G_V6", "TXV_PD_15dBm_Pout_29p5_V0", "TXV_PD_10dBm_Vout_28G_V4", "TXV_NF_Gm5dB_29p5_V0", "TXV_AMAM_12dBm_GainCompress_29p5G_V6", "TXV_OP1_Gmax_GainCompress_29p5G_V4", "TXV_GS_Gain_Dynamic_FE_29p5G_V4", "TXV_OIP3_Gmax_100M_OIP3_H_29p5G_V1", "TXV_PD_15dBm_Pout_28G_V6", "TXV_PD_15dBm_Vout_29p5_V0", "TXV_PD_15dBm_Pout_28G_V4", "TXV_NF_Gm5dB_29p5_V1", "TXV_AMPM_12dBm_PhaseDelta_29p5G_V6", "TXV_OP1_Gmax_Pout_29p5G_V5", "TXV_GS_Phase_Dynamic_COM_29p5G_V4", "TXV_OIP3_Gmax_100M_OIP3_L_29p5G_V2", "TXV_PD_15dBm_Vout_28G_V6", "TXV_PD_4dBm_Pout_29p5_V1", "TXV_PD_15dBm_Vout_28G_V4", "TXV_NF_Gm5dB_29p5_V2", "TXV_AMPM_12dBm_Pout_29p5G_V7", "TXV_OP1_Gmax_GainCompress_29p5G_V5", "TXV_GS_Phase_Dynamic_FE_29p5G_V4", "TXV_OIP3_Gmax_100M_OIP3_H_29p5G_V2", "TXV_PD_4dBm_Pout_28G_V7", "TXV_PD_4dBm_Vout_29p5_V1", "TXV_PD_4dBm_Vout_29p5_V4", "TXV_NF_Gm5dB_29p5_V3", "TXV_AMAM_12dBm_GainCompress_29p5G_V7", "TXV_OP1_Gmax_Pout_29p5G_V6", "TXV_GS_Gain_Gmax_COM127_FE127_29p5G_V5", "TXV_OIP3_Gmax_100M_OIP3_L_29p5G_V3", "TXV_PD_4dBm_Vout_28G_V7", "TXV_PD_10dBm_Pout_29p5_V1", "TXV_PD_10dBm_Pout_29p5_V4", "TXV_NF_Gm5dB_29p5_V4", "TXV_AMPM_12dBm_PhaseDelta_29p5G_V7", "TXV_OP1_Gmax_GainCompress_29p5G_V6", "TXV_GS_Gain_Dynamic_COM_29p5G_V5", "TXV_OIP3_Gmax_100M_OIP3_H_29p5G_V3", "TXV_PD_10dBm_Pout_28G_V7", "TXV_PD_10dBm_Vout_29p5_V1", "TXV_PD_10dBm_Vout_29p5_V4", "TXV_NF_Gm5dB_29p5_V5", "TXV_PAE_12dBm_Pout_29p5G_V0", "TXV_OP1_Gmax_Pout_29p5G_V7", "TXV_GS_Gain_Dynamic_FE_29p5G_V5", "TXV_OIP3_Gmax_100M_OIP3_L_29p5G_V4", "TXV_PD_10dBm_Vout_28G_V7", "TXV_PD_15dBm_Pout_29p5_V1", "TXV_PD_15dBm_Pout_29p5_V4", "TXV_NF_Gm5dB_29p5_V6", "TXV_PAE_12dBm_PAE_29p5G_V0", "TXV_OP1_Gmax_GainCompress_29p5G_V7", "TXV_GS_Phase_Dynamic_COM_29p5G_V5", "TXV_OIP3_Gmax_100M_OIP3_H_29p5G_V4", "TXV_PD_15dBm_Pout_28G_V7", "TXV_PD_15dBm_Vout_29p5_V1", "TXV_PD_15dBm_Vout_29p5_V4", "TXV_NF_Gm5dB_29p5_V7", "TXV_PAE_12dBm_Pout_29p5G_V1", "TXV_AMPM_12dBm_Pout_29p5G_V0", "TXV_GS_Phase_Dynamic_FE_29p5G_V5", "TXV_OIP3_Gmax_100M_OIP3_L_29p5G_V5", "TXV_PD_15dBm_Vout_28G_V7", "TXV_PD_4dBm_Pout_29p5_V2", "TXV_PD_4dBm_Pout_29p5_V5", "TXV_NF_Gm10dB_29p5_V0", "TXV_PAE_12dBm_PAE_29p5G_V1", "TXV_AMAM_12dBm_GainCompress_29p5G_V0", "TXV_GS_Gain_Gmax_COM127_FE127_29p5G_V6", "TXV_OIP3_Gmax_100M_OIP3_H_29p5G_V5", "TXV_GS_Gain_Gmax_COM127_FE127_29p5G_V0", "TXV_PD_4dBm_Vout_29p5_V2", "TXV_PD_4dBm_Vout_29p5_V5", "TXV_NF_Gm10dB_29p5_V1", "TXV_PAE_12dBm_Pout_29p5G_V2", "TXV_AMPM_12dBm_PhaseDelta_29p5G_V0", "TXV_GS_Gain_Dynamic_COM_29p5G_V6", "TXV_OIP3_Gmax_100M_OIP3_L_29p5G_V6", "TXV_GS_Gain_Dynamic_COM_29p5G_V0", "TXV_PD_10dBm_Pout_29p5_V2", "TXV_PD_10dBm_Pout_29p5_V5", "TXV_NF_Gm10dB_29p5_V2", "TXV_PAE_12dBm_PAE_29p5G_V2", "TXV_AMPM_12dBm_Pout_29p5G_V1", "TXV_GS_Gain_Dynamic_FE_29p5G_V6", "TXV_OIP3_Gmax_100M_OIP3_H_29p5G_V6", "TXV_GS_Gain_Dynamic_FE_29p5G_V0", "TXV_PD_10dBm_Vout_29p5_V2", "TXV_PD_10dBm_Vout_29p5_V5", "TXV_NF_Gm10dB_29p5_V3", "TXV_PAE_12dBm_Pout_29p5G_V3", "TXV_AMAM_12dBm_GainCompress_29p5G_V1", "TXV_GS_Phase_Dynamic_COM_29p5G_V6", "TXV_OIP3_Gmax_100M_OIP3_L_29p5G_V7", "TXV_GS_Phase_Dynamic_COM_29p5G_V0", "TXV_PD_15dBm_Pout_29p5_V2", "TXV_PD_15dBm_Pout_29p5_V5", "TXV_NF_Gm10dB_29p5_V4", "TXV_PAE_12dBm_PAE_29p5G_V3", "TXV_AMPM_12dBm_PhaseDelta_29p5G_V1", "TXV_GS_Phase_Dynamic_FE_29p5G_V6", "TXV_OIP3_Gmax_100M_OIP3_H_29p5G_V7", "TXV_GS_Phase_Dynamic_FE_29p5G_V0", "TXV_PD_15dBm_Vout_29p5_V2", "TXV_PD_15dBm_Vout_29p5_V5", "TXV_NF_Gm10dB_29p5_V5", "TXV_PAE_12dBm_Pout_29p5G_V4", "TXV_AMPM_12dBm_Pout_29p5G_V2", "TXV_GS_Gain_Gmax_COM127_FE127_29p5G_V7", "TXV_NF_Gmax_29p5_V0", "TXV_GS_Gain_Gmax_COM127_FE127_29p5G_V1", "TXV_PD_4dBm_Pout_29p5_V3", "TXV_PD_4dBm_Pout_29p5_V6", "TXV_NF_Gm10dB_29p5_V6", "TXV_PAE_12dBm_PAE_29p5G_V4", "TXV_AMAM_12dBm_GainCompress_29p5G_V2", "TXV_GS_Gain_Dynamic_COM_29p5G_V7", "TXV_NF_Gmax_29p5_V1", "TXV_GS_Gain_Dynamic_COM_29p5G_V1", "TXV_PD_4dBm_Vout_29p5_V3", "TXV_PD_4dBm_Vout_29p5_V6", "TXV_NF_Gm10dB_29p5_V7", "TXV_PAE_12dBm_Pout_29p5G_V5", "TXV_AMPM_12dBm_PhaseDelta_29p5G_V2", "TXV_GS_Gain_Dynamic_FE_29p5G_V7", "TXV_NF_Gmax_29p5_V2", "TXV_GS_Gain_Dynamic_FE_29p5G_V1", "TXV_PD_10dBm_Pout_29p5_V3", "TXV_PD_10dBm_Pout_29p5_V6", "TXV_PD_4dBm_Pout_29p5_V0", "TXV_PAE_12dBm_PAE_29p5G_V5", "TXV_AMPM_12dBm_Pout_29p5G_V3", "TXV_GS_Phase_Dynamic_COM_29p5G_V7", "TXV_NF_Gmax_29p5_V3", "TXV_GS_Phase_Dynamic_COM_29p5G_V1", "TXV_PD_10dBm_Vout_29p5_V3", "TXV_PD_10dBm_Vout_29p5_V6", "TXV_PD_4dBm_Vout_29p5_V0", "TXV_PAE_12dBm_Pout_29p5G_V6", "TXV_AMAM_12dBm_GainCompress_29p5G_V3", "TXV_GS_Phase_Dynamic_FE_29p5G_V7", "TXV_NF_Gmax_29p5_V4", "TXV_GS_Phase_Dynamic_FE_29p5G_V1", "TXV_PD_15dBm_Pout_29p5_V3", "TXV_PD_15dBm_Pout_29p5_V6", "TXV_PD_10dBm_Pout_29p5_V0", "TXV_PAE_12dBm_PAE_29p5G_V6", "TXV_AMPM_12dBm_PhaseDelta_29p5G_V3", "TXV_GS_Gain_Gmax_COM127_FE127_29p5G_ChannelDelta", "TXV_NF_Gmax_29p5_V5", "TXV_GS_Gain_Gmax_COM127_FE127_29p5G_V2", "TXV_PD_15dBm_Vout_29p5_V3", "TXV_PD_15dBm_Vout_29p5_V6", "TXV_PD_10dBm_Vout_29p5_V0", "TXV_PD_10dBm_Vout_29p5_V7", "RXV_GS_Gain_Dynamic_COM_24p25G_V3", "TXV_OP1_Gmax_Pout_29p5G_V0", "RXV_GS_Phase_Dynamic_COM_24p25G_V6", "TXV_GS_Gain_Dynamic_COM_29p5G_V2", "TXV_PD_4dBm_Pout_29p5_V4", "TXV_PD_4dBm_Pout_29p5_V7", "RXV_IIP3_Gmax_100M_IIP3_H_24p25G_V0", "TXV_PD_15dBm_Pout_29p5_V7", "RXV_GS_Gain_Dynamic_FE_24p25G_V3", "RXV_NF_Gmax_24p25G_VALL", "RXV_GS_Phase_Dynamic_FE_24p25G_V6", "TXV_GS_Gain_Dynamic_FE_29p5G_V2", "RXV_GS_Phase_Dynamic_COM_26p5G_V2", "TXV_PD_4dBm_Vout_29p5_V7", "RXV_IIP3_Gmax_100M_IIP3_L_24p25G_V1", "TXV_PD_15dBm_Vout_29p5_V7", "RXV_GS_Phase_Dynamic_COM_24p25G_V3", "RXV_GS_Gain_Gmax_COM127_FE127_26p5G_V0", "RXV_GS_Gain_Gmax_COM127_FE127_24p25G_V7", "RXV_GS_Gain_Dynamic_COM_26p5G_V5", "RXV_GS_Phase_Dynamic_FE_26p5G_V2", "TXV_PD_10dBm_Pout_29p5_V7", "RXV_IIP3_Gmax_100M_IIP3_H_24p25G_V1", "RXV_GS_Gain_Gmax_COM127_FE127_24p25G_V0", "RXV_GS_Phase_Dynamic_FE_24p25G_V3", "RXV_GS_Gain_Dynamic_COM_26p5G_V0", "RXV_GS_Gain_Dynamic_COM_24p25G_V7", "RXV_GS_Gain_Dynamic_FE_26p5G_V5", "RXV_GS_Gain_Gmax_COM127_FE127_26p5G_V3", "RXV_GS_Phase_Dynamic_FE_26p5G_V7", "RXV_IIP3_Gmax_100M_IIP3_L_24p25G_V2", "RXV_GS_Gain_Dynamic_COM_24p25G_V0", "RXV_GS_Gain_Gmax_COM127_FE127_24p25G_V4", "RXV_GS_Gain_Dynamic_FE_26p5G_V0", "RXV_GS_Gain_Dynamic_FE_24p25G_V7", "RXV_GS_Phase_Dynamic_COM_26p5G_V5", "RXV_GS_Gain_Dynamic_COM_26p5G_V3", "RXV_IP1_Gmax_GainCompress_-30dBm_26p5G_V0", "RXV_IIP3_Gmax_100M_IIP3_H_24p25G_V2", "RXV_GS_Gain_Dynamic_FE_24p25G_V0", "RXV_GS_Gain_Dynamic_COM_24p25G_V4", "RXV_GS_Phase_Dynamic_COM_26p5G_V0", "RXV_GS_Phase_Dynamic_COM_24p25G_V7", "RXV_GS_Phase_Dynamic_FE_26p5G_V5", "RXV_GS_Gain_Dynamic_FE_26p5G_V3", "RXV_IP1_Gmax_GainCompress_-30dBm_26p5G_V1", "RXV_IIP3_Gmax_100M_IIP3_L_24p25G_V3", "RXV_GS_Phase_Dynamic_COM_24p25G_V0", "RXV_GS_Gain_Dynamic_FE_24p25G_V4", "RXV_GS_Phase_Dynamic_FE_26p5G_V0", "RXV_GS_Phase_Dynamic_FE_24p25G_V7", "RXV_GS_Gain_Gmax_COM127_FE127_26p5G_V6", "RXV_GS_Phase_Dynamic_COM_26p5G_V3", "RXV_IP1_Gmax_GainCompress_-30dBm_26p5G_V2", "RXV_IIP3_Gmax_100M_IIP3_H_24p25G_V3", "RXV_GS_Phase_Dynamic_FE_24p25G_V0", "RXV_GS_Phase_Dynamic_COM_24p25G_V4", "RXV_GS_Gain_Gmax_COM127_FE127_26p5G_V1", "RXV_IP1_Gmax_GainCompress_-30dBm_24p25G_V0", "RXV_GS_Gain_Dynamic_COM_26p5G_V6", "RXV_GS_Phase_Dynamic_FE_26p5G_V3", "RXV_IP1_Gmax_GainCompress_-30dBm_26p5G_V3", "RXV_IIP3_Gmax_100M_IIP3_L_24p25G_V4", "RXV_GS_Gain_Gmax_COM127_FE127_24p25G_V1", "RXV_GS_Phase_Dynamic_FE_24p25G_V4", "RXV_GS_Gain_Dynamic_COM_26p5G_V1", "RXV_IP1_Gmax_GainCompress_-30dBm_24p25G_V1", "RXV_GS_Gain_Dynamic_FE_26p5G_V6", "RXV_GS_Gain_Gmax_COM127_FE127_26p5G_V4", "RXV_IP1_Gmax_GainCompress_-30dBm_26p5G_V4", "RXV_IIP3_Gmax_100M_IIP3_H_24p25G_V4", "RXV_GS_Gain_Dynamic_COM_24p25G_V1", "RXV_GS_Gain_Gmax_COM127_FE127_24p25G_V5", "RXV_GS_Gain_Dynamic_FE_26p5G_V1", "RXV_IP1_Gmax_GainCompress_-30dBm_24p25G_V2", "RXV_GS_Phase_Dynamic_COM_26p5G_V6", "RXV_GS_Gain_Dynamic_COM_26p5G_V4", "RXV_IP1_Gmax_GainCompress_-30dBm_26p5G_V5", "RXV_IIP3_Gmax_100M_IIP3_L_24p25G_V5", "RXV_GS_Gain_Dynamic_FE_24p25G_V1", "RXV_GS_Gain_Dynamic_COM_24p25G_V5", "RXV_GS_Phase_Dynamic_COM_26p5G_V1", "RXV_IP1_Gmax_GainCompress_-30dBm_24p25G_V3", "RXV_GS_Phase_Dynamic_FE_26p5G_V6", "RXV_GS_Gain_Dynamic_FE_26p5G_V4", "RXV_IP1_Gmax_GainCompress_-30dBm_26p5G_V6", "RXV_IIP3_Gmax_100M_IIP3_H_24p25G_V5", "RXV_GS_Phase_Dynamic_COM_24p25G_V1", "RXV_GS_Gain_Dynamic_FE_24p25G_V5", "RXV_GS_Phase_Dynamic_FE_26p5G_V1", "RXV_IP1_Gmax_GainCompress_-30dBm_24p25G_V4", "RXV_GS_Gain_Gmax_COM127_FE127_26p5G_V7", "RXV_GS_Phase_Dynamic_COM_26p5G_V4", "RXV_IP1_Gmax_GainCompress_-30dBm_26p5G_V7", "RXV_IIP3_Gmax_100M_IIP3_L_24p25G_V6", "RXV_GS_Phase_Dynamic_FE_24p25G_V1", "RXV_GS_Phase_Dynamic_COM_24p25G_V5", "RXV_GS_Gain_Gmax_COM127_FE127_26p5G_V2", "RXV_IP1_Gmax_GainCompress_-30dBm_24p25G_V5", "RXV_GS_Gain_Dynamic_COM_26p5G_V7", "RXV_GS_Phase_Dynamic_FE_26p5G_V4", "RXV_IIP3_Gmax_100M_IIP3_L_26p5G_V0", "RXV_IIP3_Gmax_100M_IIP3_H_24p25G_V6", "RXV_GS_Gain_Gmax_COM127_FE127_24p25G_V2", "RXV_GS_Phase_Dynamic_FE_24p25G_V5", "RXV_GS_Gain_Dynamic_COM_26p5G_V2", "RXV_IP1_Gmax_GainCompress_-30dBm_24p25G_V6", "RXV_GS_Gain_Dynamic_FE_26p5G_V7", "RXV_GS_Gain_Gmax_COM127_FE127_26p5G_V5", "RXV_IIP3_Gmax_100M_IIP3_H_26p5G_V0", "RXV_IIP3_Gmax_100M_IIP3_L_24p25G_V7", "RXV_GS_Gain_Dynamic_COM_24p25G_V2", "RXV_GS_Gain_Gmax_COM127_FE127_24p25G_V6", "RXV_GS_Gain_Dynamic_FE_26p5G_V2", "RXV_IP1_Gmax_GainCompress_-30dBm_24p25G_V7", "RXV_GS_Phase_Dynamic_COM_26p5G_V7", "RXV_IIP3_Gmax_100M_IIP3_H_26p5G_V1", "RXV_IIP3_Gmax_100M_IIP3_L_26p5G_V1", "RXV_IIP3_Gmax_100M_IIP3_H_24p25G_V7", "RXV_GS_Gain_Dynamic_FE_24p25G_V2", "RXV_GS_Gain_Dynamic_COM_24p25G_V6", "RXV_IIP3_Gmax_100M_IIP3_L_26p5G_V7", "RXV_IIP3_Gmax_100M_IIP3_L_24p25G_V0", "RXV_GS_Gain_Dynamic_FE_28G_V1", "RXV_IIP3_Gmax_100M_IIP3_L_26p5G_V2", "RXV_GS_Gain_Dynamic_FE_28G_V3", "RXV_GS_Gain_Dynamic_COM_28G_V5", "RXV_GS_Phase_Dynamic_COM_24p25G_V2", "RXV_GS_Gain_Dynamic_FE_24p25G_V6", "RXV_IIP3_Gmax_100M_IIP3_H_26p5G_V7", "RXV_GS_Gain_Gmax_COM127_FE127_28G_V7", "RXV_GS_Phase_Dynamic_COM_28G_V1", "RXV_IIP3_Gmax_100M_IIP3_H_26p5G_V2", "RXV_GS_Phase_Dynamic_COM_28G_V3", "RXV_GS_Gain_Dynamic_FE_28G_V5", "RXV_GS_Phase_Dynamic_FE_24p25G_V2", "RXV_IP1_Gmax_GainCompress_-30dBm_28G_V3", "RXV_NF_Gmax_26p5G_VALL", "RXV_GS_Gain_Dynamic_COM_28G_V7", "RXV_GS_Phase_Dynamic_FE_28G_V1", "RXV_IIP3_Gmax_100M_IIP3_L_26p5G_V3", "RXV_GS_Phase_Dynamic_FE_28G_V3", "RXV_GS_Phase_Dynamic_COM_28G_V5", "RXV_GS_Gain_Gmax_COM127_FE127_24p25G_V3", "RXV_IP1_Gmax_GainCompress_-30dBm_28G_V4", "RXV_GS_Gain_Gmax_COM127_FE127_28G_V0", "RXV_GS_Gain_Dynamic_FE_28G_V7", "RXV_GS_Gain_Gmax_COM127_FE127_28G_V2", "RXV_IIP3_Gmax_100M_IIP3_H_26p5G_V3", "RXV_GS_Gain_Gmax_COM127_FE127_28G_V4", "RXV_GS_Phase_Dynamic_FE_28G_V5", "RXV_IIP3_Gmax_100M_IIP3_H_28G_V1", "RXV_IP1_Gmax_GainCompress_-30dBm_28G_V5", "RXV_GS_Gain_Dynamic_COM_28G_V0", "RXV_GS_Phase_Dynamic_COM_28G_V7", "RXV_GS_Gain_Dynamic_COM_28G_V2", "RXV_IIP3_Gmax_100M_IIP3_L_26p5G_V4", "RXV_GS_Gain_Dynamic_COM_28G_V4", "RXV_GS_Gain_Gmax_COM127_FE127_28G_V6", "RXV_IIP3_Gmax_100M_IIP3_L_28G_V2", "RXV_IP1_Gmax_GainCompress_-30dBm_28G_V6", "RXV_GS_Gain_Dynamic_FE_28G_V0", "RXV_GS_Phase_Dynamic_FE_28G_V7", "RXV_GS_Gain_Dynamic_FE_28G_V2", "RXV_IIP3_Gmax_100M_IIP3_H_26p5G_V4", "RXV_GS_Gain_Dynamic_FE_28G_V4", "RXV_GS_Gain_Dynamic_COM_28G_V6", "RXV_IIP3_Gmax_100M_IIP3_H_28G_V2", "RXV_IP1_Gmax_GainCompress_-30dBm_28G_V7", "RXV_GS_Phase_Dynamic_COM_28G_V0", "RXV_IP1_Gmax_GainCompress_-30dBm_28G_V0", "RXV_GS_Phase_Dynamic_COM_28G_V2", "RXV_IIP3_Gmax_100M_IIP3_L_26p5G_V5", "RXV_GS_Phase_Dynamic_COM_28G_V4", "RXV_GS_Gain_Dynamic_FE_28G_V6", "RXV_IIP3_Gmax_100M_IIP3_L_28G_V3", "RXV_IIP3_Gmax_100M_IIP3_L_28G_V0", "RXV_GS_Phase_Dynamic_FE_28G_V0", "RXV_IP1_Gmax_GainCompress_-30dBm_28G_V1", "RXV_GS_Phase_Dynamic_FE_28G_V2", "RXV_IIP3_Gmax_100M_IIP3_H_26p5G_V5", "RXV_GS_Phase_Dynamic_FE_28G_V4", "RXV_GS_Phase_Dynamic_COM_28G_V6", "RXV_IIP3_Gmax_100M_IIP3_H_28G_V3", "RXV_IIP3_Gmax_100M_IIP3_H_28G_V0", "RXV_GS_Gain_Gmax_COM127_FE127_28G_V1", "RXV_IP1_Gmax_GainCompress_-30dBm_28G_V2", "RXV_GS_Gain_Gmax_COM127_FE127_28G_V3", "RXV_IIP3_Gmax_100M_IIP3_L_26p5G_V6", "RXV_GS_Gain_Gmax_COM127_FE127_28G_V5", "RXV_GS_Phase_Dynamic_FE_28G_V6", "RXV_IIP3_Gmax_100M_IIP3_L_28G_V4", "RXV_IIP3_Gmax_100M_IIP3_L_28G_V1", "RXV_GS_Gain_Dynamic_COM_28G_V1", "RXV_IIP3_Gmax_100M_IIP3_L_28G_V5", "RXV_GS_Gain_Dynamic_COM_28G_V3", "RXV_IIP3_Gmax_100M_IIP3_H_26p5G_V6", "RXV_GS_Gain_Gmax_COM127_FE127_29p5G_V0", "RXV_GS_Gain_Dynamic_COM_29p5G_V1", "RXV_IIP3_Gmax_100M_IIP3_H_28G_V4", "RXV_GS_Gain_Dynamic_FE_29p5G_V2", "RXV_GS_Gain_Dynamic_FE_29p5G_V3", "RXV_IIP3_Gmax_100M_IIP3_H_28G_V5", "RXV_GS_Gain_Dynamic_FE_29p5G_V4", "RXV_GS_Gain_Dynamic_FE_29p5G_V5", "RXV_GS_Gain_Dynamic_COM_29p5G_V0", "RXV_GS_Gain_Dynamic_FE_29p5G_V1", "RXV_GS_Gain_Dynamic_COM_29p5G_V6", "RXV_GS_Phase_Dynamic_COM_29p5G_V2", "RXV_GS_Phase_Dynamic_COM_29p5G_V3", "RXV_IIP3_Gmax_100M_IIP3_L_28G_V6", "RXV_GS_Phase_Dynamic_COM_29p5G_V4", "RXV_GS_Phase_Dynamic_COM_29p5G_V5", "RXV_GS_Gain_Dynamic_FE_29p5G_V0", "RXV_GS_Phase_Dynamic_COM_29p5G_V1", "RXV_GS_Gain_Dynamic_FE_29p5G_V6", "RXV_GS_Phase_Dynamic_FE_29p5G_V2", "RXV_GS_Phase_Dynamic_FE_29p5G_V3", "RXV_IIP3_Gmax_100M_IIP3_H_28G_V6", "RXV_GS_Phase_Dynamic_FE_29p5G_V4", "RXV_GS_Phase_Dynamic_FE_29p5G_V5", "RXV_GS_Phase_Dynamic_COM_29p5G_V0", "RXV_GS_Phase_Dynamic_FE_29p5G_V1", "RXV_GS_Phase_Dynamic_COM_29p5G_V6", "RXV_GS_Gain_Gmax_COM127_FE127_29p5G_V3", "RXV_GS_Gain_Gmax_COM127_FE127_29p5G_V4", "RXV_IIP3_Gmax_100M_IIP3_L_28G_V7", "RXV_GS_Gain_Gmax_COM127_FE127_29p5G_V5", "RXV_GS_Gain_Gmax_COM127_FE127_29p5G_V6", "RXV_GS_Phase_Dynamic_FE_29p5G_V0", "RXV_GS_Gain_Gmax_COM127_FE127_29p5G_V2", "RXV_GS_Phase_Dynamic_FE_29p5G_V6", "RXV_GS_Gain_Dynamic_COM_29p5G_V3", "RXV_GS_Gain_Dynamic_COM_29p5G_V4", "RXV_IIP3_Gmax_100M_IIP3_H_28G_V7", "RXV_GS_Gain_Dynamic_COM_29p5G_V5", "RXV_GS_Gain_Gmax_COM127_FE127_29p5G_V7", "RXV_GS_Gain_Gmax_COM127_FE127_29p5G_V1", "RXV_GS_Gain_Dynamic_COM_29p5G_V2", "RXV_GS_Phase_Dynamic_FE_29p5G_V7", "RXV_IP1_Gmax_GainCompress_-30dBm_29p5G_V3", "RXV_IP1_Gmax_GainCompress_-30dBm_29p5G_V6", "RXV_NF_Gmax_28G_VALL", "RXV_IIP3_Gmax_100M_IIP3_H_29p5G_V0", "RXV_GS_Gain_Dynamic_COM_29p5G_V7", "RXV_IIP3_Gmax_100M_IIP3_L_29p5G_V2", "RXV_IIP3_Gmax_100M_IIP3_H_29p5G_V3", "RXV_IP1_Gmax_GainCompress_-30dBm_29p5G_V0", "RXV_IP1_Gmax_GainCompress_-30dBm_29p5G_V4", "RXV_IP1_Gmax_GainCompress_-30dBm_29p5G_V7", "RXV_IIP3_Gmax_100M_IIP3_L_29p5G_V5", "RXV_IIP3_Gmax_100M_IIP3_L_29p5G_V1", "RXV_GS_Gain_Dynamic_FE_29p5G_V7", "RXV_IIP3_Gmax_100M_IIP3_H_29p5G_V2", "RXV_IIP3_Gmax_100M_IIP3_L_29p5G_V4", "RXV_IP1_Gmax_GainCompress_-30dBm_29p5G_V1", "RXV_IP1_Gmax_GainCompress_-30dBm_29p5G_V5", "RXV_IIP3_Gmax_100M_IIP3_L_29p5G_V0", "RXV_IIP3_Gmax_100M_IIP3_H_29p5G_V5", "RXV_IIP3_Gmax_100M_IIP3_H_29p5G_V1", "RXV_GS_Phase_Dynamic_COM_29p5G_V7", "RXV_IIP3_Gmax_100M_IIP3_L_29p5G_V3", "RXV_IIP3_Gmax_100M_IIP3_H_29p5G_V4", "RXV_IP1_Gmax_GainCompress_-30dBm_29p5G_V2", "RXV_IIP3_Gmax_100M_IIP3_H_29p5G_V6", "RXV_IIP3_Gmax_100M_IIP3_H_29p5G_V7", "RXV_IIP3_Gmax_100M_IIP3_L_29p5G_V6", "TXV_IF_X2_Gain_Gmax_5p2_24p25G_V1", "TXV_IF_X2_5p2_NF_Gmax_24p25G_V1", "TXV_IF_X2_5p2_NF_Gm10dB_24p25G_V1", "TXV_IF_X2_Gain_Gmax_5p2_26p5G_V1", "TXV_IF_X2_5p2_NF_Gmax_26p5G_V1", "RXV_IIP3_Gmax_100M_IIP3_L_29p5G_V7", "RXV_NF_Gmax_29p5G_VALL", "TXV_IF_X2_5p2_NF_Gm10dB_26p5G_V1", "TXV_IF_X2_5p2_OP1_Gmax_GainCompress_0dBm_24p25_V1", "TXV_IF_X2_5p2_NF_Gm5dB_24p25G_V1", "TXV_IF_X2_5p2_NF_Gm15dB_24p25G_V1", "TXV_IF_X2_5p2_OP1_Gmax_GainCompress_0dBm_26p5_V1", "TXV_IF_X2_5p2_NF_Gm5dB_26p5G_V1", "TXV_IF_X2_5p2_NF_Gm15dB_26p5G_V1", "TXV_IF_X2_Gain_Gmax_5p2_28G_V1", "TXV_IF_X2_5p2_OP1_Gmax_GainCompress_0dBm_28G_V1", "TXV_IF_X2_5p2_NF_Gmax_28G_V1", "TXV_IF_X2_5p2_NF_Gm5dB_28G_V1", "TXV_IF_X2_5p2_NF_Gm10dB_28G_V1", "TXV_IF_X2_5p2_NF_Gm15dB_28G_V1", "TXV_IF_X2_Gain_Gmax_5p2_29p5G_V1", "TXV_IF_X2_5p2_OP1_Gmax_GainCompress_0dBm_29p5_V1", "TXV_IF_X2_5p2_NF_Gmax_29p5G_V1", "TXV_IF_X2_5p2_NF_Gm5dB_29p5G_V1", "TXV_IF_X2_5p2_NF_Gm10dB_29p5G_V1", "TXV_IF_X2_5p2_NF_Gm15dB_29p5G_V1", "RXV_IF_X2_5p2_Gain_Gmax_24p25G_V1", "RXV_IF_X2_5p2_IP1_Gmax_GainCompress_24p25G_V1", "RXV_IF_X2_5p2_Gain_Gmax_26p5G_V1", "RXV_IF_X2_5p2_IP1_Gmax_GainCompress_26p5G_V1", "RXV_IF_X2_5p2_Gain_Gmax_28G_V1", "RXV_IF_X2_5p2_IP1_Gmax_GainCompress_28G_V1", "RXV_IF_X2_5p2_Gain_Gmax_29p5G_V1", "RXV_IF_X2_5p2_IP1_Gmax_GainCompress_29p5G_V1", "TXV_IF_5p2_CR_X2_CarrierLeakage_29p5G", "TXV_IF_5p2_CR_X2_Iopt_29p5G", "TXV_IF_5p2_CR_X2_Qopt_29p5G", "TXV_IF_5p2_SpurX2_T22_24p25G", "TXV_IF_5p2_SpurX2_T4m2_24p25G", "TXV_IF_5p2_SpurX2_T3m1_24p25G", "TXV_IF_5p2_SpurX2_T3m1_26p5G", "TXV_IF_5p2_SpurX2_T3m1_28G", "TXV_IF_5p2_SpurX2_CR_29p5G"]
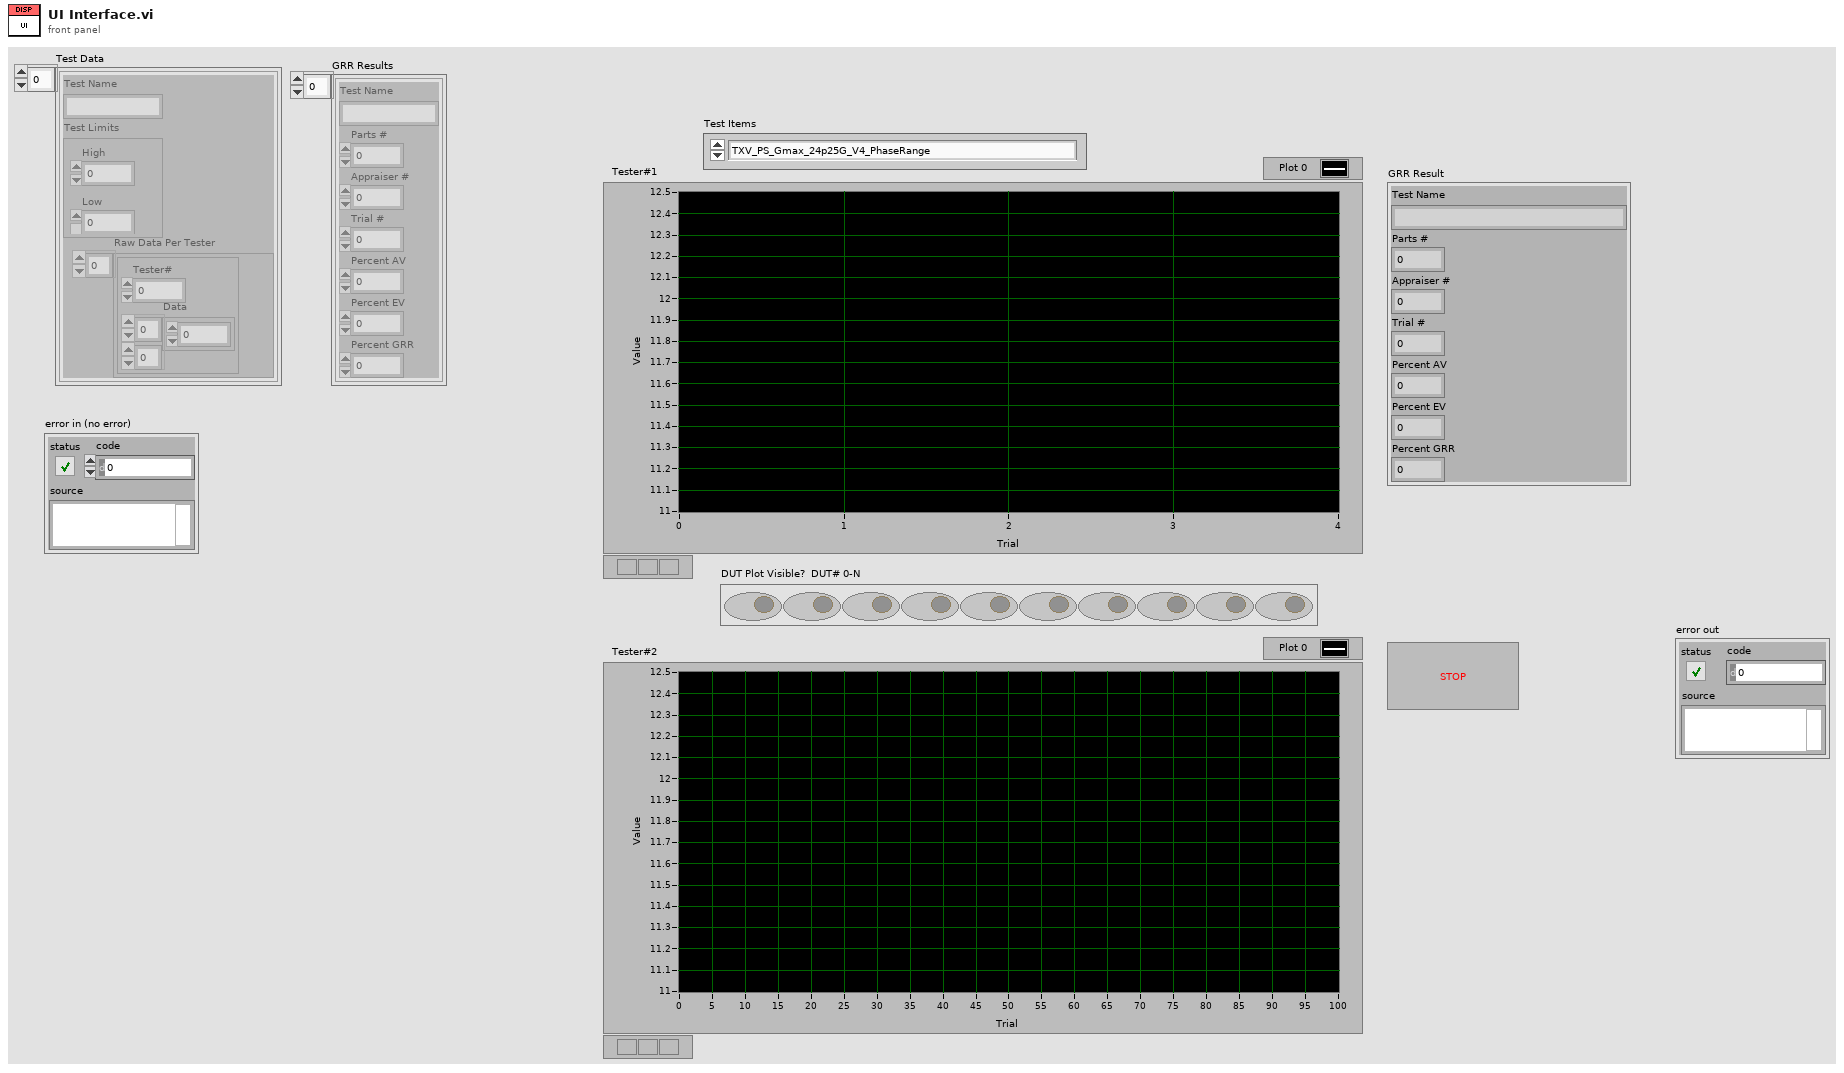
[diagram p1: front panel]
types:
  T1 = typedef "Result Data Mgr.lvclass/GRR Result.ctl" = cluster{"Test Name":string, "Parts #":u8, "Appraiser #":u8, "Trial #":u8, "Percent AV":dbl, "Percent EV":dbl, "Percent GRR":dbl}
  T2 = typedef "TestDataMgr.lvclass/Test Data All.ctl" = cluster{"Test Name":string, "Test Limits":T3, "Raw Data Per Tester":T4[]}
  T3 = typedef "TestDataMgr.lvclass/Test Limits.ctl" = cluster{"High":dbl, "Low":dbl}
  T4 = typedef "TestDataMgr.lvclass/Test Raw Data.ctl" = cluster{"Data":dbl[][], "Tester#":u8}
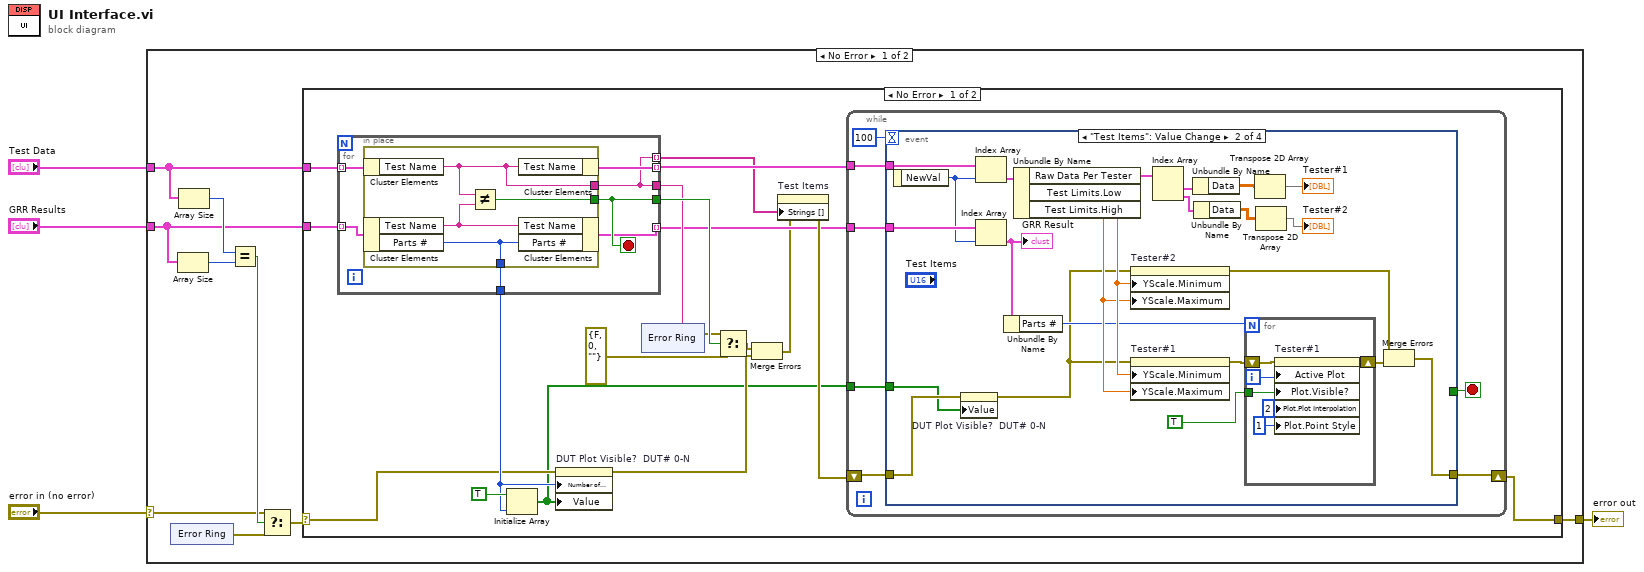
[diagram p0: block diagram]
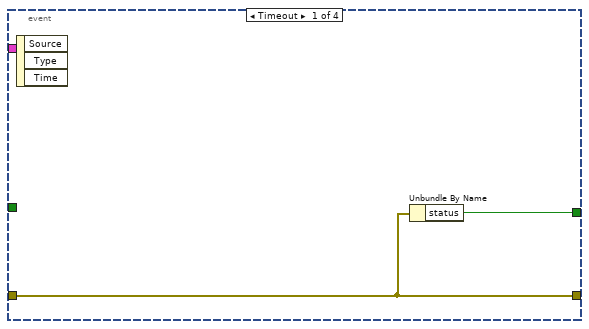
[diagram p2: hidden frame]
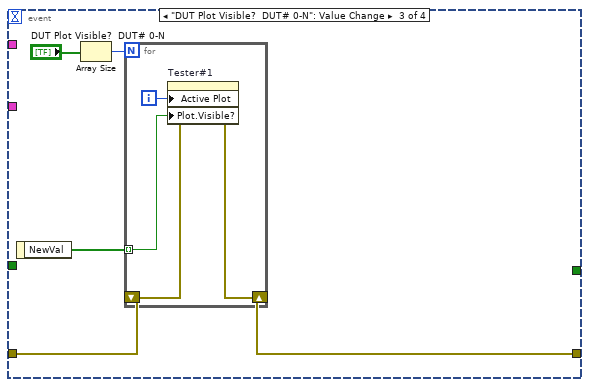
[diagram p3: hidden frame]
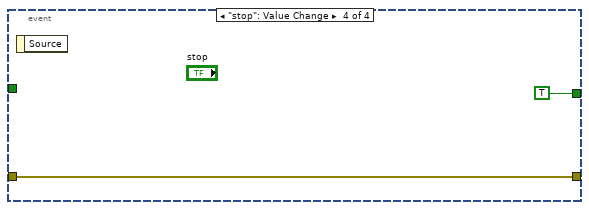
[diagram p4: hidden frame]
diagram:
  n1 = case shown="No Error" "error in (no error)" {
    selector: "error in (no error)" -> [w10 w105]
    tunnel: "Test Data" -> [w7 _]
    tunnel: "GRR Results" -> [w6 _]
    tunnel: [w5 w105] -> w3
    frame No Error {
      n2 = xnode "Error Ring"() -> ("error out"=w9:errorcluster)
      n3 = Array Size(array=w6) -> (size(s)=w13:i32)
      n4 = Array Size(array=w7) -> (size(s)=w12:i32)
      n5 = Equal?(x=w12, y=w13) -> (x = y?=w11:bool)
      n6 = Select(t=w10, s=w11, f=w9) -> (s? t:f=w8:errorcluster)
      n7 = case shown="No Error" w8 {
        selector: w8 -> [w19 w99]
        tunnel: w7 -> [w31 _]
        tunnel: w6 -> [w30 _]
        tunnel: [w22 w99] -> w5
        frame No Error {
          n8 = for {
            tunnel: w31 -> [w94] mode=indexing
            tunnel: w30 -> [w93] mode=indexing
            tunnel: [w89] -> w27
            tunnel: [w92] -> w29
            tunnel: [w91] -> w25 mode=indexing
            tunnel: [w90] -> w24 mode=indexing
            tunnel: [w89] -> w23 mode=indexing
            tunnel: [w88] -> w20
            stop <- w92 stop-if-true
            n9 = in-place {
              in-place-border: [w97] -> w92
              in-place-border: [w96] -> w89
              in-place-border: [w95] -> w88
              n10 = in-place-cluster #1(w94) -> ("Test Name"=w96:string)
              n11 = in-place-cluster #2(w93) -> ("Test Name"=w98:string, "Parts #"=w95:u8)
              n12 = Not Equal?(x=w96, y=w98) -> (x != y?=w97:bool)
              n13 = in-place-cluster #1("Test Name"=w96) -> (w91:T2)
              n14 = in-place-cluster #2("Test Name"=w98, "Parts #"=w95) -> (w90:T1)
            }
          }
          n15 = Initialize Array(TRUE, w20) -> (w14:bool[])
          n16 = property on="DUT Plot Visible?  DUT# 0-N" class="Arr (strict)"(error in=w19, "Number of Columns"=w20, "Value"=w14) -> (error out=w16:errorcluster)  [unwired: 1 in, 1 out]
          n17 = xnode "Error Ring"("parameter 0"=w27) -> ("error out"=w28:errorcluster)
          n18 = Select(t=w28, s=w29, f=errorcluster {"status"=FALSE, "code"=0, "source"=""}) -> (s? t:f=w17:errorcluster)
          n19 = Merge Errors(w17, w16) -> (w15:errorcluster)
          n20 = property on="Test Items" class="Ring (strict)"(error in=w15, "Strings []"=w23) -> (error out=w26:errorcluster)  [unwired: 1 in, 1 out]
          n21 = while {
            tunnel: w25 -> [w36]
            tunnel: w24 -> [w35]
            shift-right: [w34] -> w22
            shift-left: w26 -> [w38]
            tunnel: w14 -> [w32]
            stop <- w33 stop-if-true
            n22 = event shown="[1] \"Test Items\": Value Change" {
              selector: _ -> [_ _ _ _]
              dyn-events: _ -> [_ _ _ _]
              timeout: 100 -> [_ _ _ _]
              tunnel: w38 -> [w40 w43 w72 w80]
              tunnel: w36 -> [_ w63 _ _]
              tunnel: w35 -> [_ w62 _ _]
              tunnel: [w40 w49 w70 w80] -> w34
              tunnel: [w39 _ _ TRUE ("status")] -> w33
              tunnel: w32 -> [_ w41 _ _]
              event Timeout {
                n23 = event-data() -> ()  [unwired: 1 in, 3 out]
                n24 = Unbundle By Name(w40) -> ("status"=w39:bool)
              }
              event "Test Items": Value Change {
                n25 = event-data() -> ("NewVal"=w61:u16)  [unwired: 1 in]
                n26 = property on="DUT Plot Visible?  DUT# 0-N" class="Arr (strict)"(error in=w43, "Value"=w41) -> (error out=w42:errorcluster)  [unwired: 1 in, 1 out]
                n27 = Index Array(array=w63, index=w61) -> (element=w60:T2)
                n28 = Index Array(array=w62, index=w61) -> (element=w46:T1)
                "GRR Result" <- w46
                n29 = Unbundle By Name(w46) -> ("Parts #"=w44:u8)
                n30 = Unbundle By Name(w60) -> ("Raw Data Per Tester"=w53:T4[], "Test Limits.Low"=w52:dbl, "Test Limits.High"=w51:dbl)
                n31 = property on="Tester#2" class="WFGraph (strict)"(error in=w42, "YScale.Minimum"=w52, "YScale.Maximum"=w51) -> (error out=w50:errorcluster)  [unwired: 1 in, 1 out]
                n32 = property on="Tester#1" class="WFGraph (strict)"(error in=w42, "YScale.Minimum"=w52, "YScale.Maximum"=w51) -> (error out=w48:errorcluster)  [unwired: 1 in, 1 out]
                n33 = Index Array(array=w53) -> (element #1=w59:T4, element #2=w58:T4)  [unwired: 2 in]
                n34 = Unbundle By Name(w59) -> ("Data"=w57:dbl[][])
                n35 = Unbundle By Name(w58) -> ("Data"=w56:dbl[][])
                n36 = for {
                  N: w44 -> [_]
                  shift-right: [w68] -> w47
                  shift-left: w48 -> [w69]
                  tunnel: TRUE ("Plot.Visible") -> [w67]
                  i -> [w66]
                  n37 = property on="Tester#1" class="WFGraph (strict)"(error in=w69, "Active Plot"=w66, "Plot.Visible?"=w67, "Plot.Plot Interpolation"=u8 2, "Plot.Point Style"=u8 1) -> (error out=w68:errorcluster)  [unwired: 1 in, 1 out]
                }
                n38 = Transpose 2D Array(2D array=w57) -> (transposed array=→"Tester#1":dbl[][])
                n39 = Transpose 2D Array(2D array=w56) -> (transposed array=→"Tester#2":dbl[][])
                n40 = Merge Errors(w50, w47) -> (w49:errorcluster)
              }
              event "DUT Plot Visible?  DUT# 0-N": Value Change {
                n41 = event-data() -> ("NewVal"=w71:bool[])  [unwired: 1 in]
                n42 = Array Size(array="DUT Plot Visible?  DUT# 0-N") -> (size(s)=w73:i32)
                n43 = for {
                  N: w73 -> [_]
                  tunnel: w71 -> [w76] mode=indexing
                  shift-right: [w75] -> w70
                  shift-left: w72 -> [w78]
                  i -> [w77]
                  n44 = property on="Tester#1" class="WFGraph (strict)"(error in=w78, "Active Plot"=w77, "Plot.Visible?"=w76) -> (error out=w75:errorcluster)  [unwired: 1 in, 1 out]
                }
              }
              event "stop": Value Change {
                n45 = event-data() -> ()  [unwired: 1 in, 1 out]
              }
            }
          }
        }
        frame Error {
        }
      }
    }
    frame Error {
    }
  }
  "error out" <- w3
